vi "1_WF_Anomaly_Detection(Training).vi"() -> ()   [LabVIEW 2020]
doc: "Demonstrates the usage of Deep Learning Toolkit for solving hand written digit recognition problem with multilayer perceptron (MLP).\nDataset: MNIST http://yann.lecun.com/exdb/mnist/\nRequirements: Deep Learning Toolkit for LabVIEW"
uses:
  <vilib>/Ngene/Deep Learning Toolkit/Toolkit/NN_Layers/Layers/FC/NN_Layer_Create(FC).vi
  <vilib>/Ngene/Deep Learning Toolkit/Toolkit/Deep_Learning_Toolkit_by_Ngene.lvlib
  <vilib>/Ngene/Deep Learning Toolkit/Toolkit/NN_Activations/Controls/NN_Activation_Type.ctl
  <vilib>/Ngene/Deep Learning Toolkit/Toolkit/NN_Layers/Controls/NN_Layer_Weight_Init_Type.ctl
  <vilib>/Ngene/Deep Learning Toolkit/Toolkit/NN_Layers/Layers/FC/Controls/NN_Layer_Config(FC).ctl
  <vilib>/Ngene/Deep Learning Toolkit/Toolkit/NN_Layers/Controls/NN_Layer_Init_Params.ctl
  <vilib>/Ngene/Deep Learning Toolkit/Toolkit/NN_Network/Controls/NN_Save_Before_Destroy_Options.ctl
  <vilib>/Ngene/Deep Learning Toolkit/Toolkit/NN_Layers/Layers/Input/Controls/NN_Layer_Config(Input1D).ctl
  <vilib>/Ngene/Deep Learning Toolkit/Toolkit/NN_Layers/Layers/Input/Controls/Aug/NN_Input1D_Aug_Types.ctl
  <vilib>/Ngene/Deep Learning Toolkit/Toolkit/NN_Layers/Layers/Input/Controls/Aug/Aug_Distribution_Type.ctl
  <vilib>/Ngene/Deep Learning Toolkit/Toolkit/NN_Layers/Layers/Input/Controls/Aug/NN_Input1D_Aug_Config.ctl
  <vilib>/Ngene/Deep Learning Toolkit/Toolkit/NN_Layers/Layers/Input/Controls/NN_Layer_Config_Aug(Input1D).ctl
  <vilib>/Ngene/Deep Learning Toolkit/Toolkit/NN_Layers/Layers/BatchNorm/Controls/NN_BN_Params.ctl
  <vilib>/Ngene/Deep Learning Toolkit/Toolkit/NN_Data/Controls/NN_Data_type.ctl
  <vilib>/Ngene/Deep Learning Toolkit/Toolkit/NN_Train/Loss_Functions/NN_Set_Loss(MSE).vi
  <vilib>/Ngene/Deep Learning Toolkit/Toolkit/NN_Network/API/NN_Set_Input/1D/NN_Set_Input(1D_SGL_idx).vi
  <vilib>/Ngene/Deep Learning Toolkit/Toolkit/NN_Train/SubVIs/Dataset_Checks/NN_Check_Dataset(In1D_Out1D).vi
  <vilib>/Ngene/Deep Learning Toolkit/Toolkit/NN_Data/subVIs/Get_Data_Vals/2D/NN_Data_Get_ValByRef(2D_SGL_idx).vi
  <vilib>/Ngene/Deep Learning Toolkit/Toolkit/NN_Data/subVIs/Dataset/NN_Variant_to_DVR/2D/NN_Data_Variant_to_DVR(2D_SGL).vi
  <vilib>/Ngene/Deep Learning Toolkit/Toolkit/NN_Layers/Layers/Input/NN_Layer_Create(Input1D).vi
  <vilib>/Ngene/Deep Learning Toolkit/Toolkit/NN_Train/Controls/NN_Train_Params.ctl
  <vilib>/Ngene/Deep Learning Toolkit/Toolkit/NN_Train/Controls/NN_Train_Optimizer.ctl
  <vilib>/Ngene/Deep Learning Toolkit/Toolkit/NN_Train/Controls/NN_Train_Data_Sampling.ctl
  <vilib>/Ngene/Deep Learning Toolkit/Toolkit/NN_Train/Controls/NN_LR_Policy_Cfg.ctl
  <vilib>/Ngene/Deep Learning Toolkit/Toolkit/NN_Train/Controls/NN_LR_Policy_Type.ctl
  <vilib>/Ngene/Deep Learning Toolkit/Toolkit/NN_Train/Controls/NN_Train_Session_Data.ctl
  <vilib>/Ngene/Deep Learning Toolkit/Toolkit/NN_Network/Controls/NN_Device.ctl
panel:
  in  "Normal/Abnormal":bool
  in  "Validation(Abnormal) dataset path":path=path "D:/working/Anomaly Detection/Validation/Abnormal"
  in  "Validation(Normal) dataset path":path=path "D:/working/Anomaly Detection/Validation/Normal"
  in  "Train(Normal) dataset path":path=path "D:/working/Anomaly Detection/Train/Normal"
  out "Anomaly Score":sgl[](graph)=[0.047715902, 0.0025810003, 0.03008771, 0.04086566, 0.019934595, 0.02072841, 0.0149457455, 0.08990282, 0.04745221, 0.015019298, 0.018292785, 0.0050038695, 0.002488315, 0.0028447509, 0.004739225, 0.010417283, 0.0008608699, 0.025781095, 0.041939437, 0.002177596, 0.030179203, 0.0060115457, 0.04382831, 0.008363903, 0.035011828, 0.017032087, 0.029628694, 0.021256387, 0.014783263, 0.0030152798, 0.04009849, 0.015383124, 0.02279979, 0.09830141, 0.05799836, 0.0716297, 0.059378862, 0.07344711, 0.014608145, 0.045564353, 0.03737527, 0.0685637, 0.011108518, 0.055187643, 0.06568843, 0.046909392, 0.08090776, 0.029245019, 0.07148337, 0.11219716, 0.044215024, 0.11832294, 0.08198395, 0.053228647, 0.07091209, 0.0885334, 0.058026433, 0.017299205, 0.10348101, 0.013669521, 0.03535597, 0.10071623, 0.071124, 0.0867627, 0.055037647, 0.07809419, 0.063929304, 0.09206711, 0.03949539, 0.06335864, 0.025317574, 0.044594247, 0.08671756, 0.04539752, 0.06144145, 0.08248095, 0.05114709, 0.05862011, 0.06603286, 0.09389028, 0.06712115, 0.020853668, 0.08240548, 0.014169961, 0.06548619, 0.04012689, 0.02436462, 0.01728043, 0.069858015, 0.051284492, 0.035428643, 0.034920096, 0.05079633, 0.013650358, 0.038449407, 0.072441995, 0.01997292, 0.01657921, 0.079446375, 0.047097266, 0.10212082, 0.069970906, 0.03263557, 0.011909723, 0.02189827, 0.055327, 0.04355514, 0.028891742, 0.01913482, 0.058493435, 0.011139393, 0.01143378, 0.014839649, 0.040195167, 0.009240687, 0.010291278, 0.015378237, 0.016267061, 0.003749907, 0.02106136, 0.016822755, 0.0022764802, 0.0017397404, 0.020062983, 0.018739343, 0.05193913, 0.03168899, 0.020839095, 0.027151585, 0.03018701, 0.08075106, 0.056096375, 0.016889036, 0.014461637, 0.007615447, 0.096250534, 0.031947672, 0.045618832, 0.02684486, 0.032492936, 0.10601777, 0.045766532, 0.04348582, 0.042030573, 0.023353934, 0.05998373, 0.0366776, 0.06305903, 0.056597233, 0.063667536, 0.07347995, 0.07877654, 0.06869215, 0.030154347, 0.026351511, 0.07292321, 0.048226207, 0.06911442, 0.061527252, 0.049791813, 0.022428751, 0.09012309, 0.05610344, 0.04756078, 0.10269791, 0.044763505, 0.037158728, 0.0665781, 0.0756947, 0.09361246, 0.06363701, 0.008728512, 0.09949104, 0.07122695, 0.05130792, 0.09140627, 0.12899953, 0.076311275, 0.0602033, 0.03847994, 0.08415595, 0.026524559, 0.040219232, 0.029841065, 0.019441903, 0.027596563, 0.036504567, 0.068241, 0.040837616, 0.060942143, 0.07109749, 0.087195516, 0.055428743, 0.034413338, 0.060889006, 0.01936555, 0.07435298, 0.021365583, 0.038746476, 0.010917008, 0.096129775, 0.0073545575, 0.018815577, 0.015265167, 0.00051921606, 0.0005454421, 0.032729268, 0.07274318, 0.021330833, 0.003663838, 0.024942815, 0.02740407, 0.022603393, 0.0010912418, 0.004935682, 0.015568614, 0.02322489, 0.061240435, 0.03903711, 0.018600821, 0.029732943, 0.010967314, 0.0050938725, 0.015568972, 0.01381135, 0.0060880184, 0.051804125, 0.029231787, 0.043424904, 0.037299037, 0.031615973, 0.025720596, 0.010907292, 0.06714964, 0.0299322, 0.028302133, 0.037716627, 0.07724661, 0.07695699, 0.061065674, 0.04031396, 0.03340876, 0.020174026, 0.021361232, 0.031035602, 2.5510788e-05, 0.06611949, 0.065181196, 0.07024175, 0.07379931, 0.02338016, 0.025277913, 0.0055065155, 0.060077965, 0.05007845, 0.0006414056, 0.008725882, 0.06499711, 0.06931132, 0.09831908, 0.03877449, 0.06776312, 0.054472774, 0.063369066, 0.10040367, 0.038953096, 0.0059058666, 0.079504, 0.06579788, 0.08279285, 0.06685422, 0.040227413, 0.07007362, 0.023337401, 0.029114477, 0.057252172, 0.059272468, 0.03851404, 0.042808067, 0.045550957, 0.025526091, 0.034937397, 0.07195531, 0.025468454, 0.048014283, 0.052251175, 0.04166785, 0.056905627, 0.033443123, 0.09689638, 0.04616779, 0.0030216873, 0.031601846, 0.0032452047, 0.06213686, 0.009469092, 0.009331822, 0.017578483, 0.0055819154, 0.039248586, 0.019154549, 0.013008833, 0.014207482, 0.011167049, 0.0221982, 0.008898735, 0.017789245, 0.0074011683, 0.007955074, 0.06367123, 0.04036933, 5.1558018e-05, 0.0071540475, 0.00062155724, 0.06258881, 0.037797153, 0.0061836243, 0.02504605, 0.049601614, 0.026825964, 0.04358393, 0.02686894, 0.029046476, 0.022919714, 0.020350873, 0.035184503, 0.044800043, 0.04430455, 0.044790626, 0.050938547, 0.02782923, 0.017992377, 0.008529186, 0.06955361, 0.014567971, 0.06049311, 0.051484466, 0.07520199, 0.026690483, 0.0007273555, 0.06006384, 0.035137475, 0.023988783, 0.04264629, 0.08530253, 0.013767004, 0.012914777, 0.02451408, 0.026325583, 0.032611787, 0.064222634, 0.024199843, 0.039880395, 0.103859544, 0.014500618, 0.04841256, 0.067343056, 0.0752911, 0.06550676, 0.08130729, 0.01691103, 0.064186096, 0.030386895, 0.06907874, 0.0639095, 0.0068291724, 0.055976212, 0.021428794, 0.0060348213, 0.07295263, 0.0783522, 0.05744706, 0.0002130419, 0.040154114, 0.04585275, 0.05419886, 0.028338127, 0.08427024, 0.0041232556, 0.0687013, 0.017003741, 0.000155963, 0.07071774, 0.09512867, 0.062037416, 0.011336282, 0.040281475, 0.029887855, 0.014321253, 0.022058427, 0.014215231, 0.0059666634, 0.029912263, 0.015743941, 0.04712984, 0.016992033, 0.014030933, 0.06364295, 0.014751732, 0.03660071, 0.014532447, 0.015742123, 0.022628248, 0.018354058, 0.03808874, 0.0030311942, 0.010040998, 0.028261065, 0.017250061, 0.026884079, 0.011155605, 0.008957207, 0.008917749, 0.010064304, 0.00031030178, 0.0019487143, 0.023727417, 0.0073465705, 0.06893164, 0.04322183, 0.018407762, 0.014500916, 0.009902358, 0.03955823, 0.044618487, 0.0144174695, 0.010543764, 0.059186935, 0.04768741, 0.0011883378, 0.017390609, 0.004475951, 0.0034196973, 0.020150483, 0.017876565, 0.0039088726, 0.07626921, 0.0007389188, 0.01714021, 0.05900985, 0.033863187, 0.014671922, 0.046043932, 0.010165513, 0.011143982, 0.052004993, 0.014238179, 0.03479117, 0.025385618, 0.008669257, 0.005661547, 0.031372964, 0.054353297, 0.05981648, 0.014439642, 0.044225216, 0.009740174, 0.06296551, 0.014956772, 0.06298792, 0.05486363, 0.028136253, 0.03962207, 0.039901912, 0.058602363, 0.041279078, 0.040257484, 0.013936877, 0.07086399, 0.02723828, 0.03215918, 0.044406503, 0.02660507, 0.09844187, 0.015807092, 0.0022975206, 0.018990919, 0.03249289, 0.052985646, 0.0596376, 0.018778317, 0.05455137, 0.038281374, 0.022315275, 0.053559072, 0.046947896, 0.0041363873, 0.022759922, 0.040063687, 0.02208151, 0.024711475, 0.0038131028, 0.0016301423, 0.019919693, 0.073530674, 0.012975574, 0.0032351613, 0.033508807, 0.022399366, 0.0033747852, 0.028906435, 0.034864515, 0.00394547, 0.0149511695, 0.00368917, 0.02648884, 0.0371809, 0.017273486, 0.00536865, 0.04249835, 0.024990976, 0.014424562, 0.0037795901, 0.035405636, 0.054773033, 0.023358285, 0.023425102, 0.0194816, 0.0021141171, 0.033955276, 0.031220973, 0.016408503, 0.04635465, 0.053446114, 0.03696829, 0.03385341, 0.014172077, 0.0044620037, 0.02061069, 0.07261884, 0.008972824, 0.015659451, 0.008246541, 0.0019729137, 0.0710991, 0.05038321, 0.0028544068, 0.037355185, 0.03963381, 0.014549613, 0.0038695335, 0.03834486, 0.0026820302, 0.029096782, 0.03855908, 0.041218698, 0.02275443, 0.04536414, 0.066978574, 0.051580906, 0.0017378926, 0.025789797, 0.040744185, 0.009256244, 0.034905314, 0.03186083, 0.05465746, 0.08973676, 0.04353434, 0.022286654, 0.0051453114, 0.00048309565, 0.03697884, 0.04100603, 0.006838441, 0.035681367, 0.012636542, 0.045780897, 0.04042518, 0.0755156, 0.0016447008, 0.0059679747, 0.0072202384, 0.01067698, 0.0070519447, 0.038136035, 0.0004273653, 0.06682205, 0.01769942, 0.06582381, 0.029339477, 0.01768677, 0.0058039725, 0.023210868, 0.023157693, 0.0009084493, 0.016897243, 0.005831221, 0.031396866, 0.01948181, 0.04044591, 0.017842405, 0.013730571, 0.021805942, 0.01105006, 0.02152425, 0.065292746, 0.021284014, 0.024479747, 0.008365303, 0.023296893, 0.0356026, 0.0074109435, 9.998679e-05, 0.0040650666, 0.06386435, 0.016895354, 0.017855644, 0.011718214, 0.003956735, 0.062547326, 0.054714262, 0.014458597, 0.002638638, 0.010711074, 0.038244665, 0.007031977, 0.017196178, 0.044457376, 0.03590107, 0.009813726, 0.019953907, 0.047487378, 0.019844353, 0.034417152, 0.018498003, 0.014561772, 0.06384802, 0.031535804, 0.011589706, 0.001119554, 0.04682505, 0.056577682, 0.00937444, 0.0059499145, 0.0002413392, 0.03447455, 0.027209401, 0.00010806322, 0.029770195, 0.0073183775, 0.04158777, 0.011110187, 0.026478708, 0.0050107837, 0.04203552, 0.012228727, 0.007688701, 0.004582584, 0.025569081, 0.042006016, 0.032153547, 0.020944834, 0.05830443, 0.024040341, 0.04531777, 0.005422652, 0.055900514, 0.06162244, 0.048154175, 0.037574172, 0.009326458, 0.028306842, 0.039817393, 0.025396824, 0.00022929907, 0.019289196, 0.037306607, 0.0028678775, 0.02366358, 0.072078794, 0.032467306, 0.0025970936, 0.017390937, 0.010368198, 0.002228558, 0.022588015, 0.017153263, 0.03150198, 0.0044680536, 0.008227289, 0.005346477, 0.0020497143, 0.041761637, 0.009586662, 0.042886183, 0.035135306, 0.016337283, 0.043457747, 0.03837393, 0.051611952, 0.021941999, 0.014178699, 0.037345707, 0.014388442, 0.018260948, 0.05853848, 0.029040098, 0.025413066, 0.012405887, 0.022361755, 0.026380628, 0.018216312, 0.0015644729, 0.020917326, 0.019475996, 0.024011612, 0.017211854, 0.021681547, 0.015715957, 0.027698696, 0.011981189, 0.03608662, 0.0057917833, 0.009307146, 0.009901524, 0.0032221675, 0.037121236, 0.006166756, 0.0054784417, 0.011930764, 0.0014172792, 0.05286801, 0.044288397, 0.011786461, 0.005430579, 0.019859195, 0.013941109, 0.034538627, 0.0028657913, 0.047690094, 0.0014411211, 0.06301719, 0.01045537, 0.036057293, 0.0025453568, 0.009298801, 0.028163493, 0.02333951, 0.0074952245, 0.0109013915, 0.037617683, 0.021433711, 0.015725017, 0.02000618, 0.018161058, 0.0010209084, 0.004538834, 0.01497376, 0.008681357, 0.03325498, 0.012607813, 0.025254905, 0.046028495, 0.020547867, 0.027874947, 0.019095242, 0.0067641735, 0.029079497, 0.0304721, 0.03780067, 0.042236805, 0.03193754, 0.009736061, 0.045875132, 0.019194245, 0.020226657, 0.012554288, 0.024856985, 0.0032795072, 0.008099079, 0.016595662, 0.009702802, 0.043530464, 0.055282056, 0.008933961, 0.06304589, 0.025927782, 0.0014396906, 0.02054578, 0.024381757, 0.037120134, 0.057779104, 0.032738894, 0.043530256, 0.01557222, 0.025099546, 0.01085031, 0.003905654, 0.012544721, 0.048828557, 0.02195388, 0.020418592, 0.005827032, 0.040778756, 0.014163524, 0.015930746, 0.029816426, 0.0112039, 0.020876735, 0.015639842, 0.046031654, 0.006152123, 0.009709865, 0.015743494, 0.02742067, 0.014137089, 0.019241929, 0.041894466, 0.0380778, 0.017151564, 0.028223097, 0.0073495805, 0.02557528, 0.05750835, 0.052480698, 0.023915052, 0.018465817, 0.0607692, 0.04103142, 0.0051792264, 0.062756956, 0.0017514229, 0.047276914, 0.03923863, 0.0414052, 0.02587217, 0.0129439235, 0.0024460554, 0.030288875, 0.006010711, 0.012355745, 0.020411193, 0.021352828, 0.015683293, 0.00407207, 0.016973317, 0.03465146, 0.054066658, 0.016430616, 0.00036644936, 0.06764871, 0.0023283362, 0.026587725, 0.010902405, 0.015266538, 0.019437015, 0.029160678, 0.01953113, 0.0073716044, 0.048199713, 0.008838415, 0.008901656, 0.011385918, 0.030213773, 0.022456944, 0.016247928, 0.014270544, 0.008595407, 0.061956167, 0.0069187284, 0.017821848, 0.039972365, 0.0042414665, 0.05832219, 0.054510415, 0.026431322, 0.035200596, 0.02948153, 0.06208718, 0.032461464, 0.038664818, 0.0013316274, 0.02666688, 0.009301305, 0.0017058849, 0.0044255257, 0.010630608, 0.0064505935, 0.03288746, 0.029383928, 0.0012662113, 0.074050486, 0.061786264, 0.04708299, 0.028854996, 0.07325849, 0.03170407, 0.01122728, 0.021617055, 0.027222857, 0.027592361, 0.07195831, 0.030459575, 0.033628687, 0.021496147, 0.04374882, 0.018187447, 0.036165297, 0.023571942, 0.021791894, 0.0085014105, 0.0108578205, 0.05386503, 0.05539906, 0.0006233007, 0.0037605017, 0.0017763972, 0.022153169, 0.062341124, 0.044531137, 0.068103254, 0.06815606, 0.004120916, 0.022712916, 0.016933113, 0.025369227, 0.04291123, 0.040973663, 0.0039020777, 0.059156835, 0.011050403, 0.06237316, 0.03736663, 0.044977903, 0.015730858, 0.014122486, 0.016065955, 0.029520154, 0.03648597, 0.07051659, 0.0013179779, 0.02324748, 0.065591395, 0.025277019, 0.004920244, 0.022859454, 0.00853914, 0.03705609, 0.019424379, 0.025880516, 0.026400805, 0.0066967607, 0.0113399625, 0.022522569, 0.024003327, 0.017210007, 0.024513185, 0.043397844, 0.014945388, 0.005337, 0.02035439, 0.005132377, 0.034187138, 0.0031021833, 0.037469983, 0.0021530986, 0.0030584931, 0.00672853, 0.013904095, 0.026868641, 0.006538272, 0.028280377, 0.01350528, 0.028854728, 0.027126312, 0.0120072365, 0.05255574, 0.0076737404, 0.036070883, 0.006802559, 0.01700586, 0.031392276, 0.016890705, 0.03442079, 0.018255591, 0.051992595, 0.0022095442, 0.03269446, 0.022119522, 0.050598025, 0.04284787, 0.016165614, 0.046081275, 0.04473442, 0.037802935, 0.03842947, 0.06306109, 0.02220431, 0.028944224, 0.0045770705, 0.042494506, 0.008256197, 0.046750844, 0.0036908686, 0.02311422, 0.00077693164, 0.0039515197, 0.018653229, 0.07726545, 0.040283788, 0.059524216, 0.009495227, 0.047083277, 0.020730667, 0.049935937, 0.012333117, 0.05908279, 0.06908634, 0.06223628, 0.033225983, 0.004655093, 0.05483687, 0.056556523, 0.016717672, 0.02827838, 0.071347386, 0.01589346, 0.06992328, 0.0028676689, 0.0745683, 0.08355194, 0.040931225, 0.06754261, 0.021474183, 0.027969003, 0.0076584816, 0.047234952, 0.019856632, 0.01673466, 0.048998177, 0.027508855, 0.002669096, 0.024096966, 0.023823977, 0.030286014, 0.053969204, 0.01939392, 0.023516238, 0.031034708, 0.038506985, 0.047025442, 0.018635392, 0.034413576, 0.012740314, 0.050352156, 0.018050969, 0.041873693, 0.0032143593, 0.00026267767, 0.045363843, 0.011178076, 0.020819843, 0.020995736, 0.019217253, 0.024541855, 0.021695912, 0.042124867, 0.039527237, 0.013458908, 0.022761524, 0.042527378, 0.018703818, 0.016821265, 0.007864118, 0.018794596, 0.002880156, 0.011899173, 0.03275305, 0.051254213, 0.019226491, 0.01218617, 0.02842462, 0.06131518, 0.037252605, 0.0028996468, 0.004270494, 0.023361921, 0.011644244, 0.0009986758, 0.011639357, 0.022646487, 0.030133486, 0.0023872852, 0.05259055, 0.02781564, 0.019533455, 0.011627108, 0.05079347, 0.03150606, 0.006302446, 0.0426268, 0.058501363, 0.041143566, 0.05102235, 0.017350227, 0.044205993, 0.059088513, 0.016211674, 0.013123974, 0.10360771, 0.06259384, 0.07653545, 0.054447174, 0.06402078, 0.05027257, 0.010026, 0.0012903884, 0.017136708, 0.031048805, 0.02365224, 0.028259784, 0.034087062, 0.09500918, 0.10728651, 0.08586332, 0.15200752, 0.11835763, 0.16687855, 0.17173398, 0.19207877, 0.24995285, 0.19854617, 0.1764394, 0.21960711, 0.20500982, 0.24628907, 0.25381434, 0.28048664, 0.27028018, 0.2936979, 0.31636304, 0.34905374, 0.2980923, 0.33609152, 0.34724927, 0.36034995, 0.32336485, 0.3780651, 0.39284462, 0.34902, 0.36514992, 0.36266762, 0.39584345, 0.41756094, 0.40966296, 0.41349822, 0.38569427, 0.40935284, 0.41609186, 0.450463, 0.41314453, 0.4588943, 0.4453857, 0.4970355, 0.40337288, 0.482355, 0.4416746, 0.42152506, 0.44260156, 0.47098666, 0.5108878, 0.48012918, 0.44878733, 0.4477948, 0.42475057, 0.45093548, 0.45039457, 0.47215348, 0.44049102, 0.40422547, 0.47909123, 0.3841099, 0.44589847, 0.38989443, 0.37071013, 0.38811028, 0.34597635, 0.43548524, 0.3414498, 0.3586625, 0.34691823, 0.32170552, 0.3432048, 0.3056975, 0.32426786, 0.34024483, 0.2951817, 0.2671197, 0.26881975, 0.26968446, 0.2301977, 0.20990345, 0.2044313, 0.23516709, 0.22842091, 0.19398198, 0.15870875, 0.18524614, 0.15944, 0.12737198, 0.14472875, 0.13780338, 0.11759119, 0.11801046, 0.12755883, 0.08333115, 0.04292041, 0.0053507686, 0.090944454, 0.011543207, 0.019948155, 0.005117163, 0.052084804, 0.019741476, 0.054212824, 0.04441881, 0.13271424, 0.07727906, 0.07064524, 0.11240524, 0.11976227, 0.15400401, 0.17976153, 0.11758286, 0.17170012, 0.16568577, 0.16813141, 0.22549754, 0.20982617, 0.30876273, 0.29224867, 0.29248106, 0.25594628, 0.30639195, 0.25497818, 0.29515803, 0.33552432, 0.31921124, 0.3067137, 0.24702018, 0.31533587, 0.3658582, 0.36704057, 0.35608792, 0.37667185, 0.39209074, 0.38716066, 0.36213583, 0.37161422, 0.39183903, 0.40344232, 0.45020974, 0.40157467, 0.43283337, 0.45464092, 0.4650002, 0.4078399, 0.44429886, 0.39547884, 0.43432665, 0.42246765, 0.37123108, 0.45490205, 0.47389477, 0.41789138, 0.4096067, 0.42737395, 0.40034485, 0.46786267, 0.4371156, 0.4394366, 0.42294914, 0.40482736, 0.45386964, 0.41958004, 0.41875392, 0.43256062, 0.41303563, 0.39032292, 0.35937828, 0.39335245, 0.37966162, 0.3207494, 0.34534585, 0.31439143, 0.35419393, 0.35136044, 0.2714697, 0.3071317, 0.3122294, 0.3169033, 0.25213546, 0.17343307, 0.28683865, 0.21691835, 0.2296286, 0.24889404, 0.16115963, 0.22275573, 0.21703765, 0.16188416, 0.20319314, 0.1351986, 0.06677234, 0.1281872, 0.121130824, 0.095688134, 0.1242291, 0.053609952, 0.076433584, 0.05226974, 0.019035295, 0.04608327, 0.051075764, 0.041780293, 0.002134502, 0.016285017, 0.014686391, 0.035825074, 0.07825789, 0.08928537, 0.0548864, 0.06708887, 0.12011245, 0.15190464, 0.18970129, 0.18528613, 0.14642143, 0.17787713, 0.19936293, 0.18542993, 0.20661956, 0.19919503, 0.20683569, 0.2254808, 0.23557454, 0.26535833, 0.278089, 0.33645636, 0.32736862, 0.33491045, 0.39516985, 0.3846696, 0.3192271, 0.35689765, 0.38337123, 0.36489803, 0.37651008, 0.3748414, 0.393134, 0.39248073, 0.4201432, 0.3958295, 0.40006888, 0.44861025, 0.42295724, 0.42890185, 0.43160933, 0.45493543, 0.42765456, 0.45452338, 0.4304362, 0.3685441, 0.40631235, 0.40755337, 0.44663572, 0.42920858, 0.4233718, 0.38530934, 0.4663105, 0.44680423, 0.41557652, 0.4176917, 0.41162497, 0.39407736, 0.3614812, 0.4195885, 0.43954504, 0.398023, 0.42228526, 0.35042423, 0.41396052, 0.387394, 0.34367543, 0.39515483, 0.3506348, 0.31913853, 0.2936976, 0.31444108, 0.33919525, 0.34410495, 0.30420256, 0.31221074, 0.29192054, 0.26789325, 0.28812188, 0.24974829, 0.28794038, 0.19300196, 0.18817458, 0.22424757, 0.21683434, 0.17423075, 0.18689865, 0.15911564, 0.1098187, 0.1137068, 0.1202703, 0.122633025, 0.0856407, 0.08053285, 0.061647743, 0.057097957, 0.04922293, 0.05724816, 0.001163342, 0.003945347, 0.013643123, 0.010027081, 0.0108757615, 0.08470482, 0.08373572, 0.07757519, 0.11199492, 0.12700078, 0.095326394, 0.101403326, 0.11915606, 0.12910521, 0.14894515, 0.14079827, 0.18173847, 0.21615872, 0.21829468, 0.20423907, 0.26865637, 0.2269032, 0.2324276, 0.28228277, 0.24751759, 0.24826968, 0.24185771, 0.32894927, 0.27344245, 0.280459, 0.3615561, 0.30175394, 0.41692477, 0.39269507, 0.4353841, 0.4031086, 0.3606316, 0.32949835, 0.35444605, 0.3942849, 0.36237657, 0.4052484, 0.37975264, 0.4004873, 0.40951306, 0.37155914, 0.39112228, 0.4454437, 0.39413953, 0.50151587, 0.41670054, 0.40516222, 0.42869157, 0.3719684, 0.45527446, 0.4354626, 0.3855487, 0.37958026, 0.44542348, 0.4463405, 0.41590822, 0.4122483, 0.369613, 0.43961388, 0.4128676, 0.41172755, 0.34417838, 0.35851038, 0.39117116, 0.39790213, 0.37138748, 0.35669726, 0.3281142, 0.2862726, 0.37756056, 0.33414364, 0.34650546, 0.29717416, 0.27725822, 0.3376863, 0.2689234, 0.2523632, 0.29676956, 0.23450476, 0.23432785, 0.19972146, 0.15833294, 0.19368213, 0.17604354, 0.19002718, 0.19075039, 0.19072005, 0.16317034, 0.125684, 0.1071043, 0.10264088, 0.15311924, 0.094702795, 0.104200944, 0.06759892, 0.044868685, 0.04457221, 0.044390526, 0.041599587, 0.009926207, 0.016707115, 0.041193113, 0.0037209839, 0.0052166283, 0.098388866, 0.061579272, 0.068443745, 0.14088993, 0.095683336, 0.12377456, 0.11309707, 0.10020709, 0.1467542, 0.14300224, 0.21611425, 0.19595557, 0.22386393, 0.23261929, 0.26708806, 0.21489549, 0.265872, 0.28999883, 0.2594192, 0.30382723, 0.27976763, 0.29174453, 0.3503322, 0.29209417, 0.32555664, 0.33462924, 0.3401587, 0.3462242, 0.35842872, 0.34520954, 0.38784915, 0.35780674, 0.04020959, 0.08372176, 0.0776189, 0.060139894, 0.097709894, 0.08003843, 0.07797986, 0.051816642, 0.047575057, 0.069582105, 0.0674656, 0.07808864, 0.05615127, 0.06218505, 0.017017365, 0.06487441, 0.0010330677, 0.038105726, 0.011226773, 0.021775484, 0.07733595, 0.063058734, 0.053465366, 0.027271926, 0.046481013, 0.09432882, 0.038227737, 0.07192367, 0.06956929, 0.051414967, 0.02923429, 0.046415985, 0.06561458, 0.05245942, 0.018404424, 0.051792502, 0.049830258, 0.033891737, 0.07359338, 0.005530715, 0.07115489, 0.029260635, 0.041643023, 0.018743515, 0.015555918, 0.011587262, 0.03343004, 0.03461951, 0.021687478, 0.03833261, 0.037670672, 0.007627785, 0.03832051, 0.009793431, 0.014735758, 0.016792923, 0.024642855, 0.025508285, 0.030881107, 0.06366445, 0.030663773, 0.03541994, 0.02178897, 0.036904372, 0.05318751, 0.0036119688, 0.010256409, 0.009168476, 0.015120845, 0.0044179335, 0.03668298, 0.047770068, 0.0040861666, 0.015399441, 0.026566625, 0.014979377, 0.012833685, 0.03807065, 0.015267134, 0.014687568, 0.015760303, 0.07911828, 0.0031440854, 0.0021149516, 0.056374997, 0.05004096, 0.012219667, 0.10929704, 0.057184935, 0.0428949, 0.012614727, 0.08175272, 0.031056225, 0.04383546, 0.06013894, 0.05104482, 0.04815787, 0.031544924, 0.06282681, 0.082015455, 0.06751734, 0.07721686, 0.06628597, 0.06583208, 0.0514853, 0.03862065, 0.028685391, 0.053161442, 0.032678843, 0.050779343, 0.026046753, 0.0924958, 0.090927124, 0.07286954, 0.08844817, 0.07528716, 0.094216466, 0.09988135, 0.08372027, 0.053912878, 0.06538564, 0.08065671, 0.10297024, 0.036806226, 0.035205603, 0.055594742, 0.076091886, 0.038747013, 0.10293436, 0.054749668, 0.045713365, 0.06508398, 0.04049349, 0.09987658, 0.015277386, 0.058148026, 0.11515927, 0.042001188, 0.0035157204, 0.062142074, 0.03937179, 0.098088264, 0.05230272, 0.05701375, 0.00393641, 0.0011408925, 0.05078411, 0.016378462, 0.04868883, 0.08481455, 0.047059596, 0.022682726, 0.026164562, 0.012143731, 0.040976644, 0.017727047, 0.09220639, 0.020482719, 0.061356157, 0.0021803975, 0.0037044883, 0.009715736, 0.052236304, 0.023337841, 0.025850326, 0.050537787, 0.013436541, 0.0055997074, 0.03712785, 0.0077945627, 0.05592349, 0.0012027062, 0.013075605, 0.020720191, 0.024010241, 0.01479581, 0.016827404, 0.030558363, 0.015124962, 0.03727129, 0.0035442412, 0.027584583, 0.006701201, 0.013814449, 0.03564605, 0.0070546865, 0.013096958, 0.011903524, 0.032976568, 0.056175947, 0.025060475, 0.031738818, 0.07220447, 0.09542501, 0.039100826, 0.07739991, 0.07337773, 0.008980811, 0.0033184886, 0.06001824, 0.055814266, 0.047296286, 0.029973269, 0.056255817, 0.059824467, 0.07536459, 0.10366714, 0.07212579, 0.039361894, 0.080531, 0.09450114, 0.063426554, 0.06223941, 0.064344406, 0.071787834, 0.108517885, 0.105495214, 0.13214654, 0.038695037, 0.0952819, 0.1254859, 0.11156398, 0.09407437, 0.09940964, 0.0997901, 0.07735628, 0.104536176, 0.10556692, 0.085997224, 0.06963652, 0.08141792, 0.07232982, 0.09118146, 0.09753454, 0.084991515, 0.084968925, 0.10546726, 0.044424415, 0.06955904, 0.091522336, 0.029014528, 0.087307155, 0.07887232, 0.10404587, 0.0933848, 0.05388266, 0.073718905, 0.05041969, 0.09238088, 0.07978207, 0.054448187, 0.087059855, 0.042691827, 0.04288125, 0.09604609, 0.04231757, 0.03933978, 0.044936746, 0.06721625, 0.09342125, 0.021906376, 0.072917074, 0.06430268, 0.0135733485, 0.009343535, 0.02072157, 0.03508824, 0.073774785, 0.01874414, 0.07625115, 0.01645761, 0.022751573, 0.01261903, 0.035796292, 0.023246653, 0.023820166, 0.043936133, 0.0059004873, 0.04301019, 0.008450046, 0.00059069693, 0.01853396, 0.027813554, 0.012709439, 0.00031155348, 0.04911858, 0.051597416, 0.025631398, 0.044952452, 0.0067074895, 0.087528706, 0.055566102, 0.05398935, 0.037686825, 0.021915913, 0.032868624, 0.0063841343, 0.06768656, 0.05494052, 0.014489055, 0.06333095, 0.057601333, 0.037834942, 0.106841505, 0.020667076, 0.06850928, 0.040855587, 0.08487272, 0.08369887, 0.1063323, 0.09598112, 0.03803581, 0.10189116, 0.042521775, 0.10309875, 0.059610844, 0.080476224, 0.08484912, 0.15615201, 0.094754815, 0.094225824, 0.061502397, 0.12885815, 0.14350593, 0.087043405, 0.08951622, 0.109604, 0.09813243, 0.095102966, 0.1376431, 0.13674217, 0.0778563, 0.11322141, 0.15300399, 0.06646758, 0.15084398, 0.12895566, 0.13326317, 0.15391177, 0.08805472, 0.090057015, 0.13663888, 0.09571856, 0.108368516, 0.09767032, 0.1320008, 0.061623037, 0.09587866, 0.05944717, 0.11934781, 0.113535106, 0.09484959, 0.111512065, 0.053406477, 0.106235206, 0.121563554, 0.15173966, 0.11799276, 0.09788814, 0.037851036, 0.0565719, 0.042096704, 0.058404982, 0.07150829, 0.06508112, 0.103627235, 0.013689637, 0.04077673, 0.0649703, 0.0070453137, 0.07181531, 0.016764373, 0.06798321, 0.016805626, 0.025288634, 0.02255059, 0.018744105, 0.022342317, 0.022829836, 0.021267038, 0.016382612, 0.0014830977, 0.03296882, 0.052188113, 0.029418543, 0.05269873, 0.06283882, 0.046594918, 0.021034151, 0.032283366, 0.029017746, 0.036972046, 0.00626719, 0.0050839484, 0.053715378, 0.03149569, 0.032604814, 0.060468495, 0.04465568, 0.06333661, 0.08593392, 0.07434738, 0.040181577, 0.09658438, 0.05523789, 0.052340746, 0.09991956, 0.08627689, 0.016836047, 0.07450122, 0.045303702, 0.06741166, 0.078064024, 0.14879322, 0.10289347, 0.08531064, 0.04481536, 0.05656004, 0.073052704, 0.04151666, 0.10891342, 0.084085464, 0.076387286, 0.102749705, 0.096190035, 0.099155486, 0.10787815, 0.10682976, 0.14352363, 0.133268, 0.10419649, 0.13158739, 0.1202181, 0.089677155, 0.08486706, 0.05886233, 0.14240217, 0.17081511, 0.18490946, 0.11767632, 0.11474764, 0.093085706, 0.06527203]
  out "Loss Chart":sgl(graph)=6.871157
  out "Input & Reconstructed Signals":sgl[][](graph)=[[-203.69182, -196.45944, -206.42105, -212.12776, -209.98431, -212.81482, -214.06697, -234.45668, -226.42854, -220.56462, -214.24974, -221.52092, -221.16281, -222.03725, -222.54259, -226.90015, -224.91339, -219.17255, -215.53453, -224.83737, -217.877, -226.08276, -213.40121, -224.96735, -213.59717, -216.4723, -226.23088, -212.33847, -211.97202, -214.08366, -201.33636, -212.25195, -211.15195, -179.20767, -185.76039, -179.36887, -178.70908, -171.73268, -182.25404, -170.74457, -168.62994, -156.8247, -171.38605, -150.91496, -143.59477, -143.30174, -130.10214, -137.22119, -121.803986, -106.51268, -117.308395, -93.7625, -96.723854, -97.62513, -87.381096, -77.151985, -78.23366, -81.768196, -54.604557, -69.67931, -57.994568, -35.828102, -36.21024, -25.736954, -26.630962, -14.377393, -11.056967, 2.416106, -3.241106, 9.206075, 7.0362177, 18.38262, 35.452217, 32.255405, 42.825947, 54.835426, 54.0353, 62.54883, 70.807884, 84.21367, 84.26908, 79.644875, 100.897316, 91.00079, 109.55669, 109.47046, 111.927505, 116.2273, 134.60593, 135.90828, 137.86287, 143.26082, 152.59111, 148.95609, 159.94786, 173.14607, 155.76651, 169.33902, 188.98714, 185.78334, 203.069, 199.43301, 194.55254, 193.17833, 188.66443, 210.55849, 211.09325, 196.82597, 210.99236, 223.07843, 209.00655, 211.09589, 212.43848, 227.56683, 221.81776, 218.5701, 218.54922, 219.29591, 223.26003, 219.82527, 221.32254, 224.81364, 225.18246, 220.54489, 229.37744, 211.93462, 215.83464, 217.4786, 214.76361, 212.59512, 199.01974, 203.01688, 210.50662, 208.68921, 207.9323, 184.01987, 196.81256, 190.41148, 191.79723, 187.0817, 165.83574, 198.66397, 173.4034, 169.67267, 169.83505, 156.7239, 157.75739, 146.86583, 143.61665, 136.87979, 129.4848, 122.93364, 119.83389, 123.56296, 118.95564, 102.018425, 101.94571, 91.17254, 86.75346, 83.56996, 83.8971, 61.17046, 63.095177, 58.665413, 38.7125, 46.13676, 41.241905, 27.461256, 18.55327, 7.53301, 8.007118, 14.225158, -14.277849, -14.454468, -16.393902, -32.977505, -48.719887, -42.794704, -45.88879, -47.395184, -65.07743, -45.234108, -67.73261, -71.96186, -75.94605, -84.38318, -93.0011, -106.85784, -106.52103, -117.346115, -126.0234, -135.64693, -134.0229, -134.7392, -146.61336, -132.87227, -160.64471, -153.20773, -162.41916, -160.78008, -186.03116, -165.75491, -167.56427, -180.06364, -180.35538, -184.6909, -196.25504, -209.69836, -200.7194, -198.08067, -208.06628, -211.53697, -213.26482, -210.50189, -211.45543, -211.06352, -211.38602, -233.3377, -229.6889, -225.98419, -229.8559, -221.04784, -223.17747, -221.38345, -222.04527, -224.13887, -237.793, -218.10437, -214.21802, -214.96823, -215.61217, -215.82706, -218.18225, -203.00409, -210.25627, -208.7275, -204.30801, -192.66081, -190.09033, -191.26424, -193.36465, -191.9019, -191.95824, -188.0733, -182.15146, -185.75388, -166.05133, -162.19652, -156.66197, -151.24817, -158.78876, -153.53331, -156.12155, -135.3413, -132.46117, -139.04605, -131.58578, -112.56069, -106.00528, -93.04342, -101.57413, -88.61685, -85.566536, -77.19142, -62.063118, -70.57126, -72.02259, -47.879044, -44.448505, -33.889717, -30.994986, -30.66542, -16.782331, -21.279024, -12.932525, 0.5405211, 7.985392, 9.72337, 17.713936, 25.09223, 27.006262, 36.224976, 51.829273, 47.39243, 59.52343, 67.260284, 71.20028, 81.57735, 82.42635, 104.13513, 98.20027, 92.634796, 107.18444, 104.82115, 126.51285, 119.87258, 121.12036, 133.33884, 133.30034, 149.33966, 149.79709, 147.35788, 158.9298, 163.00009, 159.79243, 167.54431, 178.50941, 180.09627, 180.49078, 201.7611, 180.63136, 193.66762, 198.99698, 200.54916, 188.49869, 197.32869, 210.52406, 217.45105, 225.74438, 209.32176, 207.21986, 225.80853, 213.82886, 216.73927, 218.3158, 215.71573, 214.12799, 214.48691, 214.61026, 213.37476, 218.68098, 220.56183, 222.353, 206.98712, 218.98369, 206.76166, 207.72372, 200.35153, 210.07428, 214.73456, 197.98468, 201.567, 201.60269, 194.24489, 181.12738, 195.17592, 192.02046, 185.63661, 181.60185, 176.25317, 164.58656, 169.87204, 161.7887, 141.8737, 158.75986, 145.82098, 136.23767, 129.29015, 126.35838, 117.04625, 127.22135, 110.11534, 112.46715, 97.4211, 92.66172, 103.63901, 82.32571, 84.37709, 84.728355, 59.291367, 51.515476, 50.052708, 57.06887, 41.00301, 32.91534, 24.192274, 23.67885, 3.2951412, 15.810419, -6.408311, -0.9608977, -3.8774314, -27.532257, -40.11088, -39.128983, -33.680706, -47.347557, -51.573086, -54.557102, -52.545975, -67.73166, -69.608, -84.45894, -87.53854, -101.311165, -100.318085, -99.11257, -123.7543, -118.02042, -129.02417, -129.48778, -127.981895, -142.47078, -146.96497, -156.9813, -153.6075, -160.32983, -169.50266, -163.13998, -178.29219, -178.83736, -178.09027, -182.17975, -190.57542, -191.92554, -195.8277, -193.02542, -200.07683, -221.50359, -197.22676, -205.82213, -209.15977, -212.42343, -226.21397, -207.93156, -216.61981, -224.05049, -208.51514, -212.23502, -224.6852, -220.94626, -224.28577, -226.42073, -230.19612, -220.82964, -225.57812, -205.6154, -223.02266, -217.88635, -206.63763, -211.23283, -214.15874, -204.70946, -211.16028, -208.52544, -196.3188, -202.74284, -194.93011, -194.06744, -194.71938, -192.08122, -182.31049, -172.9552, -167.80405, -174.61449, -163.14594, -166.86235, -149.52827, -156.49037, -139.92291, -136.83273, -138.20729, -129.9307, -124.58354, -114.57544, -112.97303, -107.458206, -107.77515, -88.11264, -92.58281, -85.1618, -75.98244, -73.77478, -50.053955, -63.4063, -60.168594, -49.442177, -39.721706, -28.083445, -19.766977, -22.613203, -7.3076715, -4.49247, -1.364334, 12.854177, 18.227495, 14.672733, 26.102383, 36.975285, 39.379562, 46.970757, 48.675144, 54.631233, 65.74073, 85.08736, 70.80586, 81.17644, 94.92211, 87.744156, 99.92995, 112.29755, 119.72748, 118.06692, 126.70828, 129.5254, 127.80268, 148.60342, 140.81436, 148.95152, 165.47961, 154.08217, 161.4181, 168.5329, 182.49736, 164.93446, 187.76599, 191.86203, 185.40442, 194.18738, 188.89073, 207.65303, 207.21805, 217.28513, 195.97293, 202.56761, 205.47517, 219.1613, 218.75089, 214.41342, 203.37148, 219.84653, 226.95827, 222.18083, 224.1665, 242.18379, 213.26804, 226.28506, 216.39476, 215.36787, 220.9081, 222.75131, 213.51723, 220.87631, 227.06323, 209.14583, 206.82751, 209.33893, 201.5126, 193.92514, 195.22058, 204.3029, 208.02956, 208.49861, 193.1385, 183.38274, 180.5134, 171.20221, 158.70317, 165.47176, 166.25119, 168.51488, 162.36406, 148.80508, 142.79855, 149.24123, 133.75647, 134.00723, 120.53258, 116.05795, 102.11626, 114.63473, 106.807686, 100.50714, 93.67752, 91.69247, 74.36735, 77.17743, 54.762703, 68.56786, 41.802284, 43.838524, 40.155174, 36.047047, 25.149393, 18.442154, 17.498028, 6.2646623, 2.200507, -10.895248, -5.4043655, -26.747019, -28.042177, -34.01534, -42.673428, -41.507984, -45.71418, -73.03026, -69.18816, -76.43514, -75.03233, -89.11125, -98.30463, -94.221375, -102.264, -107.26439, -129.56744, -115.945114, -121.47464, -128.46762, -137.74962, -157.33136, -160.49142, -156.11006, -158.07327, -165.05066, -176.21872, -173.28767, -171.79291, -190.66977, -192.69626, -190.2753, -196.54895, -206.51698, -193.71736, -193.33987, -200.28047, -203.86517, -225.32352, -204.8314, -211.77847, -216.9887, -207.16199, -206.50136, -223.76987, -221.292, -223.73792, -216.12611, -218.34973, -225.38594, -218.45515, -223.60359, -215.13895, -221.97356, -217.80511, -221.9974, -212.15147, -217.86511, -221.20528, -218.77982, -209.62341, -203.51855, -203.72314, -204.01324, -192.16695, -209.04968, -189.52373, -198.34143, -180.26387, -175.29062, -174.683, -173.3822, -176.08165, -167.20636, -160.12383, -158.78476, -160.26497, -150.6506, -141.2864, -144.51172, -134.24074, -117.10109, -121.087845, -122.496704, -113.18617, -109.11163, -106.13486, -93.93888, -89.00322, -94.440475, -79.567665, -72.18545, -68.96316, -61.69193, -44.457207, -45.4592, -30.747316, -25.887527, -31.520948, -10.45014, -4.7102566, 5.186868, 5.0260797, 9.882888, 22.40297, 16.706774, 31.502626, 47.889236, 47.529625, 53.379135, 56.977413, 65.846825, 73.53135, 78.05192, 80.53547, 91.42016, 97.31424, 93.11721, 100.74915, 116.08357, 120.651825, 115.99231, 125.52452, 142.5808, 138.04996, 146.9537, 147.62363, 155.81332, 150.93091, 166.12003, 170.51482, 176.38338, 177.49985, 194.84833, 196.62921, 192.66875, 194.74333, 201.56621, 196.81413, 211.32927, 205.23221, 220.24562, 211.54587, 198.47588, 218.0293, 226.09375, 218.50911, 223.03172, 228.75925, 217.59853, 222.12115, 227.25633, 216.09177, 220.21591, 221.82599, 230.16148, 229.47865, 224.15498, 222.59067, 219.1263, 223.60352, 212.0988, 221.66588, 210.65883, 203.75316, 217.57149, 203.55, 203.01715, 206.58339, 209.05908, 191.4067, 186.52783, 181.86317, 180.735, 182.22334, 169.46996, 181.00662, 166.98561, 164.50697, 168.68567, 158.70708, 150.93623, 151.82295, 144.88867, 126.832695, 118.49231, 128.38416, 105.34898, 120.942665, 109.06553, 97.78902, 90.62838, 81.33116, 70.13301, 69.66267, 60.59274, 60.822666, 52.05611, 48.755924, 43.702644, 34.909267, 19.481146, 19.211067, 12.619537, 9.401513, 13.626902, -6.279246, -13.66338, -23.715942, -26.208935, -35.250416, -40.713562, -54.727596, -48.92349, -54.789635, -67.37843, -76.66096, -73.1671, -87.65806, -99.33467, -104.658676, -105.87637, -114.53355, -115.5239, -125.89807, -139.082, -143.63538, -142.29962, -137.4082, -161.7046, -162.24754, -158.44301, -177.06168, -166.37965, -182.70645, -185.09727, -189.93726, -177.63068, -191.02654, -190.93294, -187.85068, -199.92258, -198.63461, -199.58131, -212.48468, -206.23601, -211.4227, -218.63359, -224.79636, -231.376, -223.78336, -221.19205, -238.71568, -224.2388, -218.01895, -227.49657, -221.69603, -230.26488, -218.36143, -220.43254, -226.64919, -212.59207, -225.32123, -220.1036, -218.30737, -212.10869, -212.29033, -219.89949, -217.26492, -209.3771, -194.17052, -208.0605, -207.79724, -190.80663, -196.26205, -179.92268, -177.2375, -180.13649, -174.19185, -185.63557, -159.33908, -177.71075, -156.08044, -160.24042, -149.11995, -148.48769, -145.0306, -141.22212, -132.08865, -130.66814, -115.70701, -110.78786, -111.53611, -88.06789, -85.0113, -82.30008, -80.4348, -63.297966, -67.03102, -70.61455, -56.25191, -48.426514, -54.862167, -24.250004, -27.4897, -20.009115, -15.960924, -3.9002838, -3.0750127, 7.9596715, 11.897266, 18.190056, 17.879662, 29.245876, 46.287605, 53.375774, 46.94959, 54.422523, 60.666332, 72.03676, 88.16187, 90.36747, 102.50478, 108.757454, 97.650986, 99.188896, 114.70395, 122.728615, 132.6987, 137.99367, 132.7435, 153.39764, 147.1321, 164.48956, 163.52798, 170.3947, 168.1754, 172.3494, 169.42416, 184.68484, 190.67664, 202.68398, 189.91632, 198.7794, 180.81807, 205.98648, 201.85915, 200.43373, 206.5106, 219.85347, 208.69815, 209.30867, 223.7762, 220.72722, 223.2816, 227.40543, 228.72081, 219.78961, 230.52316, 214.70453, 228.9469, 226.88087, 220.47495, 226.35178, 216.19508, 224.42451, 231.71278, 221.00325, 219.58595, 217.02516, 220.29698, 208.59154, 214.44919, 203.6927, 204.59872, 198.27487, 208.59032, 196.07826, 182.98662, 194.0817, 197.29701, 183.16739, 176.6386, 169.10585, 168.02623, 159.49901, 167.34134, 145.68178, 152.82971, 155.92667, 137.73132, 125.37648, 121.95651, 130.35976, 109.6605, 104.22374, 99.8873, 93.73692, 81.82534, 85.39096, 77.29339, 76.9015, 61.32132, 63.058514, 47.099796, 50.954193, 50.66741, 38.586464, 32.628365, 20.243225, -0.543707, 1.3718911, -9.965812, -4.918854, -20.659986, -21.29536, -35.024624, -26.80005, -50.65987, -60.02072, -64.856705, -64.614235, -64.47722, -83.000854, -89.89356, -78.78776, -95.82681, -112.40337, -105.334435, -124.30159, -114.20824, -137.17639, -145.09247, -140.6235, -152.53023, -136.4462, -153.59256, -153.75804, -168.29639, -166.5256, -170.57632, -182.87956, -182.04213, -180.40059, -177.81673, -193.39775, -198.54865, -207.83261, -202.89453, -207.00389, -211.68834, -216.36166, -221.04611, -216.63249, -222.57925, -219.53767, -230.2445, -224.17224, -231.32968, -221.70856, -223.50304, -235.28732, -222.19725, -220.36324, -230.63898, -220.74786, -219.46996, -230.087, -234.26997, -213.71347, -219.00986, -226.50276, -209.39343, -213.43108, -211.96289, -211.9526, -216.1907, -209.97124, -209.4958, -211.62073, -188.33899, -192.90564, -197.08469, -197.38191, -201.43564, -191.82063, -178.10408, -175.50491, -175.76686, -162.80537, -161.03969, -153.20654, -145.52484, -138.44797, -140.97295, -122.498276, -122.924255, -128.52802, -120.87051, -99.88957, -113.64146, -98.56741, -83.609566, -73.55968, -71.48554, -62.634636, -72.56406, -51.31056, -41.018757, -44.5892, -38.850246, -27.694149, -27.45748, -14.031494, -9.012678, 3.604988, 10.385417, 11.04624, 19.269693, 24.92719, 31.908287, 43.763462, 52.73765, 61.4191, 56.877792, 63.771236, 78.75281, 72.478195, 90.39417, 88.109146, 96.543846, 100.78109, 96.01131, 117.468925, 131.65454, 129.93428, 142.07764, 140.33061, 146.68456, 148.4432, 158.57275, 160.6325, 162.39287, 161.7471, 180.93785, 178.53804, 182.34018, 185.196, 200.07242, 192.70438, 194.67729, 210.2352, 211.40404, 216.55977, 212.91757, 211.78537, 217.2809, 219.96043, 229.75339, 226.95532, 227.97797, 222.12889, 233.0053, 223.70537, 228.38742, 216.95148, 240.15051, 221.6748, 231.67809, 236.27399, 230.73564, 222.9632, 212.42694, 218.36899, 224.21104, 222.28925, 225.41986, 216.4955, 213.7453, 205.40315, 209.40215, 214.2659, 192.2181, 210.69362, 191.06436, 199.70534, 199.02957, 189.33354, 193.68567, 166.20355, 182.53204, 171.92102, 168.01964, 167.3507, 154.99086, 156.5526, 144.41571, 132.90125, 135.5564, 134.13127, 125.323265, 116.47573, 117.312546, 113.30317, 105.49649, 88.9999, 81.25897, 80.16432, 79.0299, 63.06093, 59.414402, 57.270725, 43.2651, 34.847187, 29.618114, 19.437489, 7.0658827, 7.600524, 6.9791007, 5.6758156, -24.94667, -16.21037, -18.972443, -35.06812, -31.659647, -58.977955, -51.308926, -63.739487, -52.388584, -75.53302, -86.96514, -86.54274, -94.37706, -95.75903, -98.93723, -122.98011, -119.11197, -129.43541, -137.72845, -132.60059, -144.76172, -129.41695, -141.30032, -149.16454, -165.61288, -160.94592, -180.72523, -178.04205, -175.07417, -185.70932, -194.9487, -215.27516, -204.8794, -198.27405, -203.27026, -210.9389, -210.79875, -211.41823, -216.92145, -226.76741, -228.09259, -226.59863, -226.93384, -218.58965, -232.6621, -227.31999, -223.76617, -222.95996, -237.87843, -230.08827, -242.28506, -233.20161, -236.04778, -248.10454, -227.3035, -221.78525, -234.02606, -234.57439, -228.39024, -232.71724, -213.87296, -218.61226, -214.93523, -215.5322, -216.28143, -200.43129, -204.58078, -200.21907, -192.10545, -191.75145, -191.92252, -193.58922, -179.6754, -176.72122, -184.62015, -171.99701, -172.70607, -156.19345, -149.43349, -161.16727, -144.92839, -135.78494, -126.503204, -133.8875, -144.13606, -108.27872, -116.4196, -104.24913, -90.74542, -102.44169, -78.29863, -70.07097, -73.7078, -54.19364, -60.67234, -67.25464, -42.435074, -34.2886, -30.314848, -13.145017, -20.01361, -4.21594, 0.064736515, 2.4084709, 19.219986, 30.498182, 18.53273, 39.15228, 45.051594, 55.515266, 60.52198, 60.178104, 67.61151, 85.70726, 92.37867, 89.25301, 91.222885, 91.51169, 101.93133, 120.37886, 121.949486, 125.6729, 137.65681, 141.2113, 151.1532, 157.71944, 161.16461, 166.42212, 166.95401, 171.33864, 164.29048, 173.43152, 178.34148, 170.35924, 179.11931, 200.8255, 197.54456, 196.47092, 206.18446, 208.19757, 213.39809, 213.32782, 217.56464, 214.76566, 223.96092, 226.30348, 217.53354, 226.09027, 227.06355, 228.33377, 224.4155, 232.40291, 227.15439, 233.65532, 248.98943, 240.16502, 239.6272, 229.76744, 233.22995, 233.43077, 241.12576, 220.00548, 222.76698, 227.86163, 224.71399, 223.29001, 224.38144, 228.60452, 210.81876, 201.94919, 207.59448, 197.21153, 209.4182, 188.88947, 189.98544, 194.7179, 176.36284, 180.80763, 181.88676, 181.27258, 169.33414, 156.19315, 147.8148, 149.71138, 139.86942, 136.81906, 134.42563, 121.170746, 121.980415, 103.93431, 117.83953, 110.1181, 92.10058, 84.75976, 85.38461, 72.98432, 69.81224, 72.04351, 61.270367, 49.615128, 39.208076, 38.006233, 29.152119, 23.36454, 14.37649, 5.9464965, -6.059558, -2.919202, -12.013117, -26.31435, -30.9535, -46.050182, -33.190845, -43.503426, -55.06196, -56.88122, -63.11981, -80.56166, -88.7032, -94.04254, -101.254745, -105.85316, -116.92842, -116.22277, -116.84191, -125.20928, -137.22263, -130.16248, -148.58324, -155.17738, -151.13214, -167.15578, -174.65527, -183.39417, -169.45216, -189.73381, -194.52983, -181.30653, -201.89906, -180.01807, -191.3532, -186.62784, -199.41393, -214.4084, -226.20038, -224.53294, -218.81161, -230.30963, -223.38037, -232.37938, -230.28305, -230.51686, -241.7858, -239.01065, -227.41351, -241.16652, -216.11618, -237.19186, -240.20108, -234.55403, -247.92758, -227.45413, -231.249, -241.78831, -241.78073, -224.05835, -221.67828, -226.58203, -224.8204, -231.93288, -211.77267, -214.59178, -210.78539, -222.91719, -214.9175, -202.27892, -195.6235, -196.707, -194.71265, -195.57259, -199.6146, -171.22546, -175.16553, -165.4787, -170.11821, -167.69803, -145.75528, -154.57838, -150.63283, -131.8153, -138.59885, -130.00133, -129.90685, -130.9601, -113.59628, -108.70955, -95.99347, -86.45991, -77.10719, -74.11912, -73.27584, -68.13497, -59.12619, -37.171383, -41.11133, -28.751776, -27.456259, -22.591515, -12.58267, -2.3062742, 7.1039014, 5.05771, 21.769709, 17.953651, 37.266964, 46.98801, 34.706673, 53.620975, 62.053497, 54.506416, 75.196, 78.294106, 90.4567, 103.15029, 101.33899, 111.59946, 103.172585, 117.13067, 119.31266, 125.85138, 126.218864, 146.90509, 143.07071, 145.20027, 160.21939, 157.24147, 170.45576, 174.78131, 167.68028, 188.37741, 186.8264, 190.88898, 195.32193, 199.62619, 202.2171, 210.66972, 205.2362, 217.24638, 215.0903, 228.17322, 229.34854, 227.31358, 238.49039, 236.40921, 237.59517, 232.756, 233.17802, 239.65971, 240.11176, 243.38127, 238.59631, 240.28441, 229.68417, 240.92986, 224.87207, 233.78537, 221.22559, 228.18613, 240.32063, 235.6941, 231.71169, 223.74525, 226.43544, 235.75893, 219.89467, 225.58168, 222.37663, 214.89958, 206.69623, 207.45984, 208.4675, 201.71025, 189.69707, 193.8702, 189.31927, 181.17403, 186.14241, 162.59264, 176.19717, 161.10255, 159.03432, 148.25844, 142.21342, 135.98094, 135.46321, 129.9887, 121.125, 119.359825, 112.96096, 99.75066, 100.87692, 87.79043, 75.423416, 76.5103, 71.91428, 53.39801, 60.211464, 61.59947, 46.95931, 41.14079, 20.690647, 28.057049, 25.005003, 4.6531277, -3.9015381, -5.959566, -11.490997, -22.900303, -37.363914, -46.984818, -41.25932, -45.264133, -61.81599, -58.56495, -71.720085, -84.25696, -85.264114, -91.36501, -97.86247, -119.30839, -105.80542, -112.82759, -131.85, -136.08983, -126.90728, -161.5913, -154.3644, -156.21477, -154.22754, -175.86066, -168.4935, -176.12051, -184.59334, -186.97075, -190.59789, -190.69078, -202.03844, -210.24371, -210.36417, -216.05205, -216.78864, -219.5597, -218.99648, -218.54895, -218.5645, -226.83875, -223.84291, -230.10704, -225.85123, -243.239, -244.06252, -240.92868, -245.38756, -242.94891, -247.97195, -249.57152, -245.69287, -238.29909, -240.57254, -243.75761, -248.15286, -231.31349, -229.72934, -233.18274, -236.42204, -225.53929, -239.02425, -225.29993, -220.73122, -222.74014, -213.95844, -225.09038, -201.66656, -208.59552, -218.67822, -197.5203, -182.75623, -194.4341, -184.64923, -194.42119, -178.87265, -175.2033, -157.66473, -151.95383, -158.82819, -145.29083, -147.76532, -150.9155, -136.0943, -124.48386, -119.559494, -110.194496, -111.114395, -99.294495, -110.929535, -77.404144, -90.80548, -69.076706, -61.99092, -58.731777, -62.216713, -48.561085, -42.444077, -41.64907, -19.57523, -17.18393, -18.030684, -0.28930485, -8.861638, 11.80865, 21.378145, 29.932846, 37.682457, 42.190994, 41.321423, 59.414005, 62.18999, 56.334892, 70.90938, 84.8603, 82.87171, 94.27547, 105.75505, 104.89313, 112.34328, 118.05685, 128.87437, 140.20222, 138.4945, 145.37732, 160.60907, 171.222, 162.98419, 176.97598, 180.81065, 165.8446, 173.11644, 191.04437, 194.35542, 196.15111, 195.83359, 205.9814, 210.19788, 217.28749, 227.20012, 222.5102, 217.28685, 229.80743, 235.56027, 230.26237, 231.89746, 234.08266, 237.54907, 247.80429, 248.03885, 255.39517, 233.9268, 247.98766, 255.47662, 252.37535, 247.93785, 248.97832, 248.58961, 242.48552, 248.04869, 247.33606, 241.19934, 235.83276, 236.9803, 232.87915, 235.24355, 234.36829, 228.95796, 226.07254, 228.11215, 210.34186, 213.25417, 214.92537, 196.32349, 206.47372, 200.60936, 202.57101, 195.69235, 181.65184, 181.85254, 171.46072, 176.49141, 168.42769, 157.30757, 159.85437, 143.68604, 138.2115, 145.21106, 126.55622, 119.84155, 115.18482, 114.2919, 114.5811, 90.93753, 96.940094, 88.39264, 69.73761, 62.242447, 58.253178, 54.98118, 57.545948, 37.61859, 44.700275, 23.389826, 18.180378, 8.788568, 7.63111, -2.3408031, -20.35684, -31.904673, -29.736116, -45.362446, -39.731987, -48.338234, -59.64815, -68.355255, -71.450264, -74.80523, -69.33154, -99.98338, -99.99154, -110.86859, -107.6898, -133.08688, -131.41586, -136.79744, -138.40483, -140.13982, -148.28847, -144.14781, -166.96478, -168.94572, -157.32263, -180.55943, -183.74432, -183.56038, -204.44196, -187.8401, -203.16223, -200.36534, -214.28946, -217.60773, -226.15976, -226.79547, -215.7686, -233.73387, -221.88524, -238.5837, -230.3066, -237.2343, -239.96379, -258.51648, -244.98116, -245.8142, -238.92058, -255.80595, -259.80142, -246.25043, -247.0839, -251.66496, -248.43178, -247.22472, -256.47433, -255.29813, -239.96552, -247.01314, -254.88095, -232.43222, -250.52255, -243.10936, -241.74316, -244.05882, -225.61313, -222.97368, -231.03333, -217.85245, -217.28844, -211.12088, -215.52019, -194.54953, -198.45088, -185.38731, -195.20348, -189.24843, -179.72389, -178.9229, -159.69756, -167.09644, -165.49525, -167.21753, -153.35828, -143.01315, -122.60425, -121.09726, -111.623215, -109.297195, -106.20199, -98.41947, -101.19054, -73.12552, -73.146416, -72.47287, -51.850876, -60.675674, -40.74345, -46.31597, -27.07335, -22.389273, -15.012141, -7.138585, 9.442156, 5.560839, 12.655911, 20.788174, 31.795942, 30.247482, 57.405148, 58.66045, 70.9677, 79.88132, 82.462776, 82.8082, 91.98801, 97.44426, 105.59329, 101.45587, 110.180145, 127.85169, 128.27898, 134.30516, 146.51244, 148.23737, 158.0008, 168.70413, 170.96338, 167.80357, 186.14026, 180.7771, 184.64178, 200.38069, 201.42645, 188.60065, 206.2803, 203.11288, 211.7788, 217.69536, 237.79037, 229.65442, 228.31454, 220.99568, 226.2144, 232.33264, 226.924, 244.77922, 240.5005, 239.85294, 247.37993, 246.76561, 248.19731, 251.01076, 250.99915, 260.0457, 257.34433, 250.12717, 256.22098, 252.77235, 244.72252, 242.3681, 234.68697, 253.29652, 258.43564, 259.8983, 241.60231, 238.73944, 230.90057, 221.58528], [-192.24, -195.84, -199.2, -202.31999, -205.20001, -207.84, -210.48, -212.88, -215.04001, -216.95999, -218.64, -220.31999, -221.76001, -222.72, -223.68, -224.4, -225.12001, -225.36, -225.6, -225.36, -225.12001, -224.64, -223.92001, -222.96, -222.0, -220.56001, -219.12, -217.44, -215.52, -213.36, -210.96, -208.56, -205.68, -202.8, -199.68001, -196.56, -192.96, -189.36, -185.76, -181.68001, -177.6, -173.28, -168.72, -164.16, -159.36, -154.56, -149.52, -144.24, -138.95999, -133.44, -127.92, -122.16, -116.4, -110.4, -104.4, -98.4, -92.16, -85.920006, -79.44, -72.96, -66.48, -60.0, -53.28, -46.56, -39.84, -33.12, -26.4, -19.68, -12.72, -6.0, 0.96000004, 7.6800003, 14.64, 21.36, 28.08, 35.04, 41.76, 48.480003, 54.96, 61.68, 68.16, 74.64, 81.12, 87.600006, 93.840004, 99.840004, 106.08, 112.08, 117.84, 123.6, 129.36, 134.87999, 140.4, 145.68, 150.72, 155.76, 160.56001, 165.36, 169.92, 174.48, 178.56, 182.64, 186.72, 190.31999, 193.92001, 197.28, 200.64, 203.76, 206.40001, 209.04, 211.68001, 213.84, 216.0, 217.92, 219.6, 221.04001, 222.24, 223.2, 224.16, 224.87999, 225.36, 225.36, 225.6, 225.36, 224.87999, 224.4, 223.44, 222.48, 221.28, 219.84, 218.40001, 216.48, 214.56, 212.16, 209.76001, 207.12, 204.48, 201.36, 198.23999, 194.87999, 191.28, 187.68001, 183.84, 179.76001, 175.44, 171.12, 166.56, 162.0, 157.2, 152.16, 147.12, 141.84001, 136.32, 130.8, 125.28001, 119.52, 113.52, 107.76, 101.520004, 95.520004, 89.28, 82.8, 76.56, 70.08, 63.36, 56.88, 50.16, 43.44, 36.72, 30.0, 23.28, 16.320002, 9.599999, 2.6399999, -4.0800004, -11.04, -17.76, -24.48, -31.439999, -38.16, -44.88, -51.600002, -58.079998, -64.8, -71.28, -77.76, -84.240005, -90.48, -96.72, -102.72, -108.96, -114.71999, -120.72, -126.48, -132.0, -137.52, -142.8, -148.08, -153.12, -158.15999, -162.96, -167.52, -172.08, -176.40001, -180.48, -184.56, -188.40001, -192.24, -195.6, -198.95999, -202.08, -204.95999, -207.84, -210.23999, -212.64, -214.79999, -216.95999, -218.64, -220.31999, -221.51999, -222.72, -223.68, -224.4, -225.12001, -225.36, -225.6, -225.36, -225.12001, -224.64, -223.92001, -223.2, -222.0, -220.8, -219.12, -217.44, -215.52, -213.36, -211.2, -208.56, -205.92, -203.04001, -199.92, -196.8, -193.2, -189.6, -185.76, -181.92, -177.84, -173.52, -168.95999, -164.4, -159.6, -154.79999, -149.76001, -144.48, -139.2, -133.68, -128.15999, -122.63999, -116.64, -110.880005, -104.880005, -98.64, -92.399994, -86.159996, -79.92, -73.44, -66.96001, -60.239998, -53.760002, -47.039997, -40.32, -33.6, -26.880001, -19.92, -13.2, -6.2400002, 0.48000002, 7.44, 14.16, 20.88, 27.84, 34.559998, 41.280003, 48.0, 54.72, 61.199997, 67.92, 74.4, 80.880005, 87.12, 93.36, 99.6, 105.6, 111.6, 117.600006, 123.36, 129.12, 134.64, 139.92, 145.20001, 150.48, 155.52, 160.31999, 165.12001, 169.68001, 174.24, 178.31999, 182.4, 186.48, 190.31999, 193.68, 197.28, 200.4, 203.52, 206.40001, 209.04, 211.44, 213.84, 215.76, 217.68001, 219.36, 220.8, 222.24, 223.2, 224.16, 224.87999, 225.12001, 225.36, 225.6, 225.36, 224.87999, 224.4, 223.68, 222.48, 221.28, 220.08, 218.40001, 216.48, 214.56, 212.4, 210.0, 207.36, 204.48, 201.59999, 198.48001, 195.12001, 191.51999, 187.92, 184.08, 180.0, 175.68, 171.36, 166.8, 162.24, 157.44, 152.4, 147.36, 142.08, 136.56, 131.28, 125.520004, 119.76, 114.0, 108.0, 102.0, 95.759995, 89.52, 83.28, 76.799995, 70.32, 63.84, 57.120003, 50.64, 43.92, 37.2, 30.480001, 23.519999, 16.8, 10.08, 3.1200001, -3.8400002, -10.559999, -17.279999, -24.240002, -30.96, -37.68, -44.4, -51.12, -57.84, -64.32, -71.04, -77.28, -83.76, -90.0, -96.24, -102.479996, -108.479996, -114.479996, -120.24, -125.99999, -131.76001, -137.04, -142.56, -147.84, -152.88, -157.92, -162.72, -167.28, -171.84001, -176.16, -180.23999, -184.32, -188.15999, -192.0, -195.36, -198.72, -201.84001, -204.95999, -207.6, -210.23999, -212.64, -214.79999, -216.72, -218.64, -220.08, -221.51999, -222.72, -223.68, -224.4, -225.12001, -225.36, -225.6, -225.36, -225.12001, -224.64, -223.92001, -223.2, -222.0, -220.8, -219.36, -217.68001, -215.76, -213.59999, -211.2, -208.8, -206.16, -203.28, -200.16, -196.8, -193.44, -189.84, -186.0, -182.16, -178.08, -173.76, -169.2, -164.64, -160.08, -155.04001, -150.0, -144.95999, -139.43999, -134.16, -128.64, -122.880005, -117.12, -111.12, -105.119995, -99.119995, -92.88, -86.64, -80.159996, -73.68, -67.2, -60.719997, -54.0, -47.52, -40.8, -34.08, -27.119999, -20.4, -13.68, -6.7200003, 0.0, 6.96, 13.68, 20.640001, 27.36, 34.08, 41.04, 47.760002, 54.239998, 60.960003, 67.439995, 73.92, 80.4, 86.88, 93.12, 99.119995, 105.36, 111.36, 117.12, 123.12, 128.64, 134.16, 139.68001, 144.95999, 150.23999, 155.28, 160.08, 164.87999, 169.43999, 174.0, 178.08, 182.16, 186.24, 190.08, 193.68, 197.04, 200.16, 203.28, 206.16, 208.8, 211.44, 213.59999, 215.76, 217.68001, 219.36, 220.8, 222.0, 223.2, 224.16, 224.64, 225.12001, 225.36, 225.6, 225.36, 224.87999, 224.4, 223.68, 222.72, 221.51999, 220.08, 218.40001, 216.72, 214.79999, 212.4, 210.0, 207.6, 204.72, 201.84001, 198.72, 195.36, 191.76001, 188.15999, 184.32, 180.23999, 175.92, 171.59999, 167.28, 162.48, 157.68001, 152.64, 147.6, 142.31999, 137.04, 131.51999, 125.759995, 120.24, 114.240005, 108.24, 102.24, 96.24, 90.0, 83.52, 77.28, 70.799995, 64.32, 57.6, 50.88, 44.4, 37.440002, 30.720001, 24.0, 17.279999, 10.320001, 3.6, -3.3600001, -10.08, -17.04, -23.76, -30.720001, -37.440002, -44.16, -50.88, -57.359997, -64.079994, -70.56, -77.04, -83.52, -89.76, -96.0, -102.24, -108.24, -114.240005, -120.0, -125.759995, -131.28, -136.8, -142.31999, -147.36, -152.64, -157.44, -162.48, -167.04, -171.59999, -175.92, -180.0, -184.08, -187.92, -191.76001, -195.12001, -198.48001, -201.59999, -204.72, -207.36, -210.0, -212.4, -214.56, -216.72, -218.40001, -220.08, -221.51999, -222.72, -223.68, -224.4, -224.87999, -225.36, -225.6, -225.36, -225.12001, -224.64, -224.16, -223.2, -222.24, -220.8, -219.36, -217.68001, -215.76, -213.59999, -211.44, -209.04, -206.16, -203.28, -200.4, -197.04, -193.68, -190.08, -186.24, -182.4, -178.31999, -174.0, -169.68001, -164.87999, -160.31999, -155.28, -150.23999, -145.20001, -139.92, -134.4, -128.88, -123.12, -117.36, -111.6, -105.6, -99.36, -93.12, -86.88, -80.64, -74.159996, -67.68, -61.199997, -54.48, -47.760002, -41.04, -34.32, -27.6, -20.88, -13.92, -7.2, -0.24000001, 6.48, 13.440001, 20.16, 27.119999, 33.84, 40.56, 47.28, 54.0, 60.48, 67.2, 73.68, 80.159996, 86.4, 92.64, 98.88, 104.880005, 110.880005, 116.88, 122.63999, 128.40001, 133.92001, 139.43999, 144.72, 150.0, 155.04001, 159.84, 164.64, 169.2, 173.52, 177.84, 182.16, 186.0, 189.84, 193.44, 196.8, 200.16, 203.04001, 205.92, 208.8, 211.2, 213.59999, 215.52, 217.44, 219.12, 220.8, 222.0, 223.2, 223.92001, 224.64, 225.12001, 225.36, 225.6, 225.36, 225.12001, 224.4, 223.68, 222.72, 221.51999, 220.08, 218.64, 216.72, 214.79999, 212.64, 210.23999, 207.6, 204.95999, 202.08, 198.72, 195.6, 192.0, 188.40001, 184.56, 180.48, 176.40001, 171.84001, 167.52, 162.72, 157.92, 152.88, 147.84, 142.56, 137.28, 131.76001, 126.240005, 120.479996, 114.71999, 108.72, 102.72, 96.48, 90.24, 84.0, 77.520004, 71.04, 64.56, 58.079998, 51.36, 44.64, 37.920002, 31.199999, 24.48, 17.52, 10.8, 3.8400002, -2.88, -9.84, -16.56, -23.519999, -30.24, -36.96, -43.68, -50.399998, -57.120003, -63.6, -70.08, -76.56, -83.03999, -89.28, -95.520004, -101.76, -107.76, -113.76, -119.76, -125.28001, -131.04001, -136.56, -141.84001, -147.12, -152.4, -157.2, -162.0, -166.8, -171.36, -175.68, -180.0, -183.84, -187.92, -191.51999, -195.12001, -198.48001, -201.59999, -204.48, -207.36, -210.0, -212.4, -214.56, -216.48, -218.40001, -219.84, -221.28, -222.48, -223.68, -224.4, -224.87999, -225.36, -225.6, -225.36, -225.12001, -224.87999, -224.16, -223.2, -222.24, -221.04001, -219.36, -217.68001, -216.0, -213.84, -211.44, -209.04, -206.40001, -203.52, -200.4, -197.28, -193.92001, -190.31999, -186.48, -182.64, -178.56, -174.24, -169.92, -165.36, -160.56001, -155.52, -150.72, -145.44, -140.16, -134.64, -129.12, -123.6, -117.84, -111.84, -105.840004, -99.840004, -93.6, -87.36, -80.880005, -74.64, -67.92, -61.440002, -54.96, -48.24, -41.519997, -34.8, -28.08, -21.119999, -14.4, -7.44, -0.72, 6.2400002, 12.96, 19.92, 26.64, 33.36, 40.079998, 46.8, 53.52, 60.239998, 66.72, 73.200005, 79.68, 86.159996, 92.399994, 98.64, 104.64, 110.64, 116.64, 122.399994, 128.15999, 133.68, 139.2, 144.48, 149.52, 154.56, 159.6, 164.4, 168.95999, 173.28, 177.6, 181.92, 185.76, 189.6, 193.2, 196.56, 199.92, 203.04001, 205.92, 208.56, 210.96, 213.36, 215.52, 217.44, 219.12, 220.56001, 222.0, 222.96, 223.92001, 224.64, 225.12001, 225.36, 225.6, 225.36, 225.12001, 224.4, 223.68, 222.72, 221.51999, 220.31999, 218.64, 216.95999, 215.04001, 212.88, 210.48, 207.84, 205.20001, 202.08, 198.95999, 195.6, 192.24, 188.64, 184.79999, 180.72, 176.64, 172.08, 167.76, 162.96, 158.15999, 153.36, 148.08, 143.04001, 137.52, 132.24, 126.48, 120.72, 114.96, 108.96, 102.96, 96.96001, 90.72, 84.240005, 78.0, 71.520004, 65.04, 58.32, 51.84, 45.12, 38.399998, 31.68, 24.72, 18.0, 11.04, 4.3199997, -2.6399999, -9.360001, -16.320002, -23.04, -29.76, -36.48, -43.44, -49.920002, -56.64, -63.36, -69.840004, -76.32, -82.8, -89.04, -95.28001, -101.520004, -107.520004, -113.52, -119.28, -125.04001, -130.8, -136.32, -141.59999, -146.88, -151.92, -156.95999, -161.76001, -166.56, -171.12, -175.44, -179.76001, -183.59999, -187.68001, -191.28, -194.87999, -198.23999, -201.36, -204.24, -207.12, -209.76001, -212.16, -214.32, -216.48, -218.15999, -219.84, -221.28, -222.48, -223.44, -224.4, -224.87999, -225.36, -225.6, -225.36, -225.36, -224.87999, -224.16, -223.2, -222.24, -221.04001, -219.6, -217.92, -216.0, -213.84, -211.68001, -209.28, -206.64, -203.76, -200.64, -197.52, -194.16, -190.56001, -186.72, -182.88, -178.8, -174.48, -170.16, -165.6, -160.8, -156.0, -150.96, -145.68, -140.4, -135.12001, -129.6, -123.84, -118.08, -112.08, -106.08, -100.08, -93.840004, -87.600006, -81.36, -74.880005, -68.4, -61.92, -55.2, -48.480003, -42.0, -52.559998, -42.48, -32.4, -22.08, -11.759999, -1.6800001, 8.639999, 18.960001, 29.039999, 39.36, 49.44, 59.52, 69.6, 79.68, 89.52, 99.36, 108.96, 118.8, 128.15999, 137.76, 146.88, 156.0, 165.12001, 174.0, 182.64, 191.28, 199.43999, 207.6, 215.76, 223.44, 231.12, 238.31999, 245.52, 252.48001, 259.2, 265.68, 271.68, 277.68, 283.44, 288.96, 294.0, 299.04, 303.6, 307.91998, 312.0, 315.6, 319.2, 322.32, 325.2, 327.84003, 330.24002, 332.15997, 333.84, 335.28, 336.24, 336.96002, 337.44, 337.68, 337.44, 336.96002, 336.0, 335.04, 333.6, 331.92, 329.75998, 327.36, 324.72, 321.84, 318.72, 315.12, 311.28, 307.19998, 302.88, 298.08, 293.28, 288.0, 282.48, 276.72, 270.72, 264.48, 258.0, 251.28001, 244.56001, 237.36, 229.92, 222.24, 214.56, 206.40001, 198.23999, 189.84, 181.2, 172.56, 163.68, 154.56, 145.44, 136.07999, 126.72, 117.12, 107.520004, 97.68, 87.84, 78.0, 67.92, 57.84, 47.760002, 37.68, 27.6, 17.279999, 6.96, -3.1200001, -13.440001, -23.76, -33.84, -44.16, -54.239998, -64.32, -74.4, -84.240005, -94.079994, -103.92, -113.52, -123.12, -132.72, -142.08, -151.2, -160.31999, -169.2, -178.08, -186.72, -195.12001, -203.52, -211.44, -219.36, -227.04, -234.48, -241.92, -248.87999, -255.6, -262.32, -268.56, -274.56, -280.56, -286.08002, -291.36, -296.4, -301.2, -305.52, -309.84, -313.68002, -317.28, -320.63998, -323.76, -326.63998, -329.04, -331.2, -332.88, -334.56, -335.76, -336.72, -337.19998, -337.44, -337.44, -337.19998, -336.47998, -335.52, -334.32, -332.88, -330.96, -328.8, -326.16, -323.52002, -320.40002, -317.04, -313.44, -309.36002, -305.28, -300.72, -295.92, -290.88, -285.6, -279.84, -274.08, -267.84003, -261.6, -254.88, -248.16, -241.2, -233.76, -226.32, -218.64, -210.72, -202.56, -194.4, -185.76, -177.12, -168.48001, -159.36, -150.48, -141.12, -131.76001, -122.16, -112.560005, -102.96, -93.12, -83.28, -73.200005, -63.36, -53.28, -42.960003, -32.879997, -22.56, -12.4800005, -2.1599998, 8.160001, 18.24, 28.560001, 38.64, 48.96, 59.04, 69.119995, 78.96, 89.04, 98.88, 108.479996, 118.08, 127.68, 137.04, 146.40001, 155.52, 164.64, 173.52, 182.16, 190.8, 198.95999, 207.36, 215.28, 222.96, 230.64, 238.08, 245.04001, 251.99998, 258.72, 265.2, 271.44, 277.44, 283.19998, 288.48, 293.76, 298.56, 303.36002, 307.68, 311.76, 315.6, 318.96, 322.32, 325.2, 327.6, 330.0, 331.92, 333.6, 335.04, 336.24, 336.96002, 337.44, 337.68, 337.44, 336.96002, 336.24, 335.04, 333.6, 331.92, 330.0, 327.6, 324.96, 322.08002, 318.96, 315.36002, 311.52, 307.44, 303.12, 298.56, 293.52002, 288.24, 282.96, 277.19998, 271.2, 264.96, 258.48, 251.76001, 244.79999, 237.6, 230.4, 222.72, 214.79999, 206.88, 198.72, 190.31999, 181.92, 173.04001, 164.16, 155.28, 145.92, 136.8, 127.2, 117.84, 108.0, 98.4, 88.56, 78.479996, 68.64, 58.56, 48.480003, 38.16, 28.08, 17.76, 7.6800003, -2.6399999, -12.96, -23.04, -33.36, -43.44, -53.52, -63.6, -73.68, -83.76, -93.6, -103.44, -113.03999, -122.63999, -132.24, -141.59999, -150.72, -159.84, -168.72, -177.6, -186.24, -194.64, -203.04001, -210.96, -218.88, -226.56, -234.24, -241.44, -248.4, -255.36, -261.84, -268.08, -274.32, -280.08002, -285.6, -291.12003, -296.16, -300.96, -305.28, -309.59998, -313.44, -317.28, -320.63998, -323.52002, -326.4, -328.8, -330.96, -332.88, -334.32, -335.76, -336.47998, -337.19998, -337.44, -337.44, -337.19998, -336.72, -335.76, -334.32, -332.88, -330.96, -328.8, -326.4, -323.76, -320.63998, -317.28, -313.68002, -309.59998, -305.52, -300.96, -296.16, -291.12003, -285.84, -280.32, -274.32, -268.32, -261.84, -255.36, -248.64, -241.44, -234.24, -226.8, -219.12, -211.2, -203.04001, -194.87999, -186.24, -177.84, -168.95999, -160.08, -150.96, -141.59999, -132.24, -122.880005, -113.28, -103.44, -93.840004, -83.76, -73.92, -63.84, -53.760002, -43.68, -33.36, -23.28, -12.96, -2.88, 7.44, 17.76, 27.84, 38.16, 48.24, 58.32, 68.4, 78.479996, 88.32, 98.16, 108.0, 117.600006, 127.2, 136.56, 145.92, 155.04001, 164.16, 173.04001, 181.68001, 190.31999, 198.48001, 206.88, 214.79999, 222.48, 230.16, 237.6, 244.79999, 251.76001, 258.48, 264.96, 271.2, 276.96002, 282.72, 288.24, 293.52002, 298.32, 303.12, 205.44, 208.08, 210.72, 212.88, 215.04001, 217.2, 218.88, 220.31999, 221.76001, 222.96, 223.92001, 224.64, 225.12001, 225.36, 225.6, 225.36, 225.12001, 224.64, 223.92001, 222.96, 221.76001, 220.56001, 218.88, 217.2, 215.28, 213.12, 210.72, 208.31999, 205.68, 202.56, 199.68001, 196.32, 192.72, 189.12, 185.28, 181.44, 177.36, 173.04001, 168.48001, 163.92001, 159.12, 154.08, 149.04, 143.76, 138.48001, 133.2, 127.44, 121.68001, 115.920006, 110.159996, 103.92, 97.92, 91.68, 85.44, 78.96, 72.479996, 66.0, 59.52, 52.8, 46.32, 39.600002, 32.640003, 25.92, 19.199999, 12.24, 5.52, -1.44, -8.160001, -15.12, -21.84, -28.560001, -35.52, -42.239998, -48.96, -55.440002, -62.16, -68.64, -75.119995, -81.6, -87.84, -94.079994, -100.32, -106.56, -112.32, -118.32, -124.08, -129.84, -135.36, -140.64, -145.92, -151.2, -156.24, -161.04001, -165.6, -170.16, -174.72, -179.04, -183.12, -186.95999, -190.56001, -194.16, -197.52, -200.88, -203.76, -206.64, -209.28, -211.68001, -214.08, -216.0, -217.92, -219.6, -221.04001, -222.24, -223.44, -224.16, -224.87999, -225.36, -225.6, -225.6, -225.36, -224.87999, -224.4, -223.44, -222.48, -221.28, -219.84, -218.15999, -216.24, -214.32, -212.16, -209.76001, -207.12, -204.24, -201.12, -198.0, -194.64, -191.04001, -187.44, -183.59999, -179.52, -175.20001, -170.88, -166.32, -161.51999, -156.72, -151.68001, -146.64, -141.36, -136.07999, -130.56001, -124.799995, -119.04, -113.28, -107.28, -101.28, -95.04, -88.8, -82.32, -76.08, -69.6, -62.879997, -56.4, -49.68, -42.960003, -36.239998, -29.52, -22.8, -15.84, -9.12, -2.1599998, 4.56, 11.52, 18.24, 24.960001, 31.92, 38.64, 45.36, 52.079998, 58.56, 65.28001, 71.76, 78.24, 84.479996, 90.96, 97.2, 103.200005, 109.200005, 115.2, 120.96, 126.72, 132.48, 137.76, 143.28, 148.31999, 153.59999, 158.40001, 163.2, 168.0, 172.31999, 176.64, 180.96, 184.79999, 188.64, 192.48, 195.84, 199.2, 202.31999, 205.20001, 207.84, 210.48, 212.88, 215.04001, 216.95999, 218.64, 220.31999, 221.76001, 222.72, 223.68, 224.64, 225.12001, 225.36, 225.6, 225.36, 225.12001, 224.64, 223.92001, 222.96, 222.0, 220.56001, 219.12, 217.44, 215.52, 213.36, 210.96, 208.56, 205.68, 202.8, 199.68001, 196.56, 192.96, 189.36, 185.52, 181.68001, 177.6, 173.28, 168.72, 164.16, 159.36, 154.32, 149.28, 144.24, 138.95999, 133.44, 127.92, 122.16, 116.4, 110.4, 104.4, 98.16, 92.16, 85.68, 79.44, 72.96, 66.48, 60.0, 53.28, 46.56, 39.84, 33.12, 26.4, 19.44, 12.72, 5.76, -0.96000004, -7.92, -14.64, -21.36, -28.32, -35.04, -41.76, -48.480003, -55.2, -61.68, -68.4, -74.880005, -81.12, -87.600006, -93.840004, -100.08, -106.08, -112.08, -118.08, -123.84, -129.36, -134.87999, -140.4, -145.68, -150.72, -155.76, -160.8, -165.36, -169.92, -174.48, -178.8, -182.88, -186.72, -190.56001, -193.92001, -197.52, -200.64, -203.76, -206.64, -209.28, -211.68001, -213.84, -216.0, -217.92, -219.6, -221.04001, -222.24, -223.2, -224.16, -224.87999, -225.36, -225.36, -225.6, -225.36, -224.87999, -224.4, -223.44, -222.48, -221.28, -219.84, -218.15999, -216.48, -214.32, -212.16, -209.76001, -207.12, -204.48, -201.36, -198.23999, -194.87999, -191.28, -187.68001, -183.84, -179.76001, -175.44, -171.12, -166.56, -162.0, -156.95999, -152.16, -146.88, -141.59999, -136.32, -130.8, -125.04001, -119.52, -113.52, -107.520004, -101.520004, -95.28001, -89.04, -82.8, -76.32, -69.840004, -63.36, -56.88, -50.16, -43.44, -36.72, -30.0, -23.04, -16.320002, -9.599999, -2.6399999, 4.0800004, 11.04, 17.76, 24.72, 31.439999, 38.16, 44.88, 51.600002, 58.32, 64.8, 71.28, 77.76, 84.240005, 90.48, 96.72, 102.96, 108.96, 114.96, 120.72, 126.48, 132.0, 137.52, 142.8, 148.08, 153.12, 158.15999, 162.96, 167.52, 172.08, 176.40001, 180.72, 184.56, 188.40001, 192.24, 195.6, 198.95999, 202.08, 204.95999, 207.84, 210.23999, 212.64, 214.79999, 216.95999, 218.64, 220.31999, 221.51999, 222.72, 223.68, 224.4, 225.12001, 225.36, 225.6, 225.36, 225.12001, 224.64, 223.92001, 223.2, 222.0, 220.56001, 219.12, 217.44, 215.52, 213.36, 211.2, 208.56, 205.92]]
  in  "Stop":bool
  in  "Sample Index":i32=297 min=0 max=499
  in  "Check?":bool
  out "Train Speed (Sample/sec)":dbl=11006.39746853613 format="%#.0g"
  out "Train Speed (sec/iter)":dbl=0.011629599999992024 format="%#.4g"
  out "Train Loss":sgl=6.871157 format="%.3g"
  out "Time_Elapsed":dbl=14.061959599999994 format="%<%H:%M:%S>t"
  out "Session Data":T1={"Epochs"=12.436211, "Tot_Iter"=923, "LR"=5e-05, "LR_iter"=924}
  in  "LR Update Policy":T2={"Policy_Type"=enum."Step", "LR0"=0.0001, "k"=10.0, "WarmUp_Policy"=enum."Ramp", "WarmUp_Iter"=600, "WarmUp_Ratio"=20.0} {"WarmUp_Ratio" min=1; "WarmUp_Iter" min=1; "LR0" format="%.7f"}
  in  "Train_Params":T4={"Optimizer"=enum."Adam", "Beta_1"=0.9, "Beta_2"=0.999, "Weight Decay(L1)"=0.0, "Weight Decay(L2)"=0.0, "Data_Sampling"=enum."Random"}
  in  "NN_Device":T7=enum."GPU"
  # "Waveform Anomaly Detection - Training"
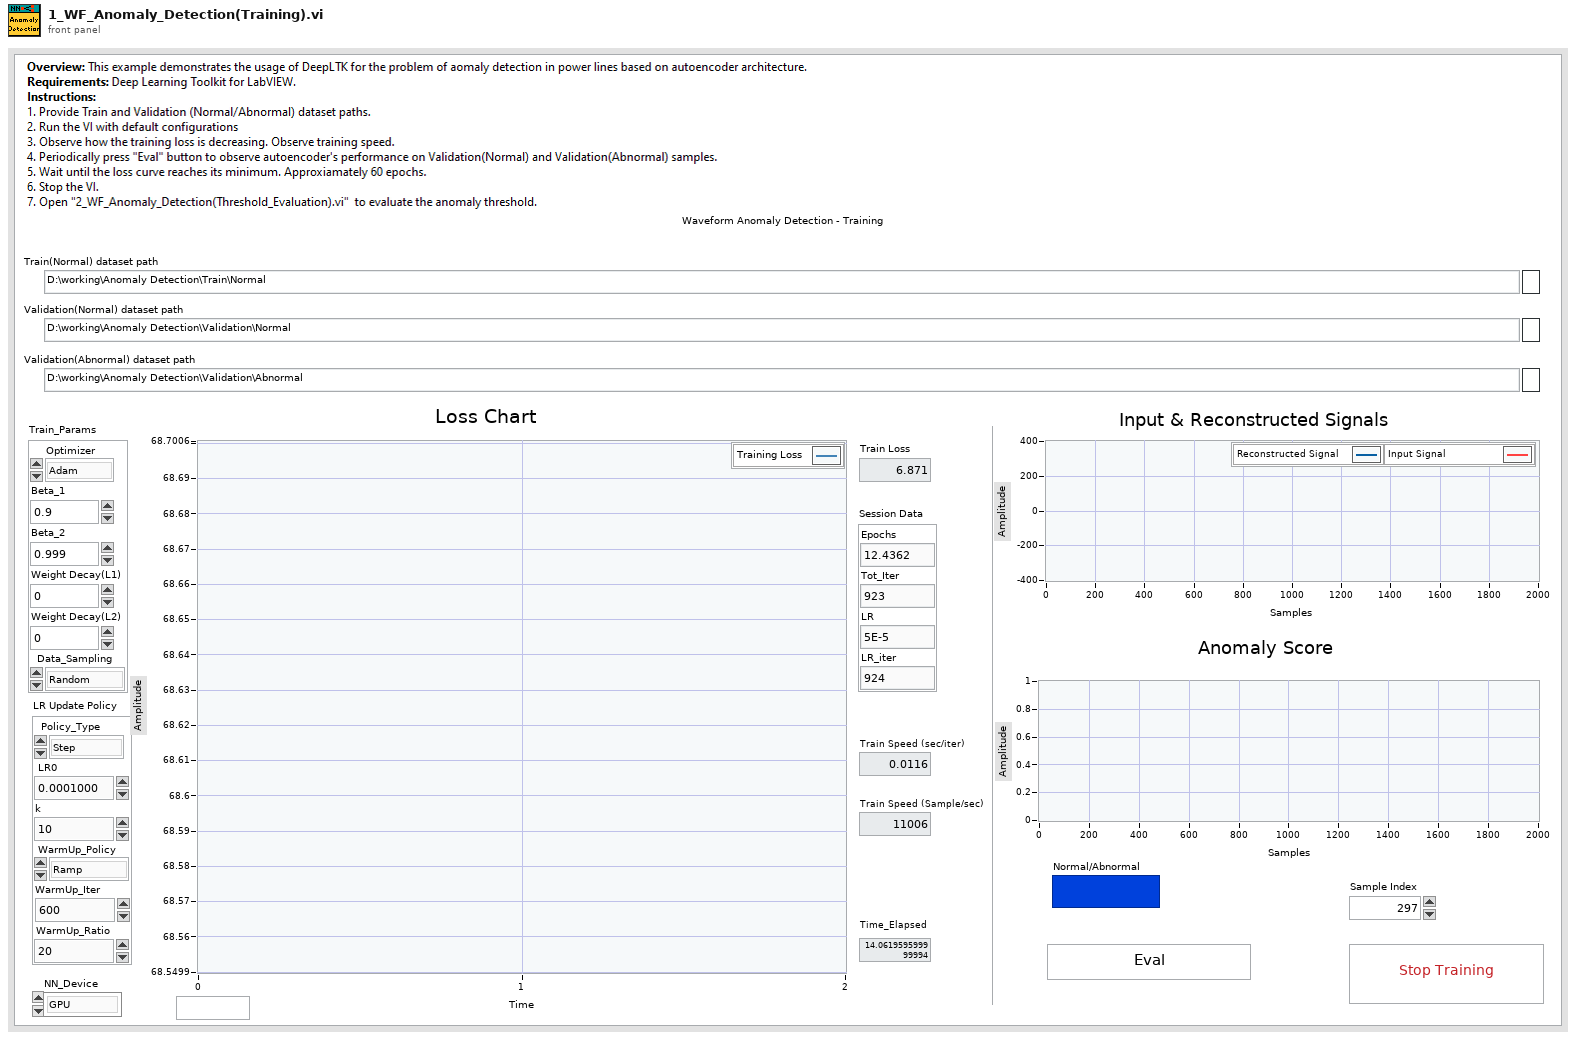
[diagram p1: front panel]
types:
  T1 = typedef "Deep_Learning_Toolkit_by_Ngene.lvlib/NN_Train_Session_Data.ctl" = cluster{"Epochs":sgl, "Tot_Iter":i32, "LR":sgl, "LR_iter":i32}
  T2 = typedef "Deep_Learning_Toolkit_by_Ngene.lvlib/NN_LR_Policy_Cfg.ctl" = cluster{"Policy_Type":T3, "LR0":dbl, "k":sgl, "WarmUp_Policy":enum16{"Step", "Ramp"}, "WarmUp_Iter":i32, "WarmUp_Ratio":sgl}
  T3 = typedef "Deep_Learning_Toolkit_by_Ngene.lvlib/NN_LR_Policy_Type.ctl" = enum16{"Manual", "Step", "Exp", "1/t"}
  T4 = typedef "Deep_Learning_Toolkit_by_Ngene.lvlib/NN_Train_Params.ctl" = cluster{"Optimizer":T5, "Beta_1":sgl, "Beta_2":sgl, "Weight Decay(L1)":sgl, "Weight Decay(L2)":sgl, "Data_Sampling":T6}
  T5 = typedef "Deep_Learning_Toolkit_by_Ngene.lvlib/NN_Train_Optimizer.ctl" = enum16{"SGD", "Adam", "Adagrad", "Adadelta", "RMSProp", "Nesterov"}
  T6 = typedef "Deep_Learning_Toolkit_by_Ngene.lvlib/NN_Train_Data_Sampling.ctl" = enum16{"Random", "Sequential"}
  T7 = typedef "Deep_Learning_Toolkit_by_Ngene.lvlib/NN_Device.ctl" = enum16{"CPU", "GPU"}
  T8 = typedef "Deep_Learning_Toolkit_by_Ngene.lvlib/NN_Layer_Config_Aug(Input1D).ctl" = T9[]
  T9 = typedef "Deep_Learning_Toolkit_by_Ngene.lvlib/NN_Input1D_Aug_Config.ctl" = cluster{"Aug Type(1D)":T10, "Aug Value":sgl, "Distribution":T11}
  T10 = typedef "Deep_Learning_Toolkit_by_Ngene.lvlib/NN_Input1D_Aug_Types.ctl" = enum16{"Add_Noise", "Mult_Noise", "Shift", "Scale"}
  T11 = typedef "Deep_Learning_Toolkit_by_Ngene.lvlib/Aug_Distribution_Type.ctl" = enum16{"Uniform", "Gaussian"}
  T12 = typedef "Deep_Learning_Toolkit_by_Ngene.lvlib/NN_Layer_Config(FC).ctl" = cluster{"Name":string, "Size":i32, "BN":bool, "BN_Params":T13, "Activation":T14, "Has Bias?":bool, "Init_Params":T15, "Custom_Params":string}
  T13 = typedef "Deep_Learning_Toolkit_by_Ngene.lvlib/NN_BN_Params.ctl" = cluster{"epsilon":sgl, "momentum":sgl}
  T14 = typedef "Deep_Learning_Toolkit_by_Ngene.lvlib/NN_Activation_Type.ctl" = enum16{"Sigmoid", "ReLU", "LReLU", "ReLU6", "tanh", "Swish", "Mish", "None"}
  T15 = typedef "Deep_Learning_Toolkit_by_Ngene.lvlib/NN_Layer_Init_Params.ctl" = cluster{"Init_Type":T16, "Value":sgl}
  T16 = typedef "Deep_Learning_Toolkit_by_Ngene.lvlib/NN_Layer_Weight_Init_Type.ctl" = enum16{"Const", "Uniform", "Gaussian", "Xavier"}
  T17 = typedef "Deep_Learning_Toolkit_by_Ngene.lvlib/NN_Layer_Config(Input1D).ctl" = cluster{"Name":string, "Size":i32, "Data_Type":T18, "Shift":sgl, "Scale":sgl}
  T18 = typedef "Deep_Learning_Toolkit_by_Ngene.lvlib/NN_Data_type.ctl" = enum16{"I8", "U8", "I16", "U16", "U32 ARGB", "SGL"}
  T19 = typedef "Deep_Learning_Toolkit_by_Ngene.lvlib/NN_Save_Before_Destroy_Options.ctl" = cluster{"CFG?":bool, "Weights?":bool, "Render?":bool}
  T20 = typedef "Deep_Learning_Toolkit_by_Ngene.lvlib/NN_DataSet(In1D_Out1D).ctl" = cluster{"Inputs Ref.":variant, "Outputs Ref.":T21, "Dims_In":i32, "Dataset_Size":i32, "Dims_Out":i32, "Labels":string[], "File Paths":path[]}
  T21 = typedef "Deep_Learning_Toolkit_by_Ngene.lvlib/NN_Data_ref(2D_SGL).ctl" = refnum<data-value>
  T22 = typedef "Deep_Learning_Toolkit_by_Ngene.lvlib/NN.ctl" = cluster{"Name":string, "No of Layers":i32, "mBatch":i32, "Layers":T23[], "Dimty":T24, "Dims_In":T25, "Dims_Out":T25, "Working_Dir":path, "Train?":bool, "Train_Params":T4, "LR_Update_Policy":T2, "Session Data":T1, "Ground_truth":T26, "NNg_hdls":T27, "NN_Device":T7, "GPU Id":i32, "Labels":string[], "Receptive Field":T28[], "Loss_Type":T29, "Loss_Cfg_Prms":variant, "NNG_WS":T30}
  T23 = typedef "Deep_Learning_Toolkit_by_Ngene.lvlib/NN_Layer_ref.ctl" = refnum<data-value>
  T24 = typedef "Deep_Learning_Toolkit_by_Ngene.lvlib/NN_In_Out_Dim-ty.ctl" = enum8{"In1D_Out1D", "In3D_Out1D", "In3D_Out3D", "In3D_OutBBox"}
  T25 = typedef "Deep_Learning_Toolkit_by_Ngene.lvlib/NN_Dims(C,H,W).ctl" = cluster{"C":i32, "H":i32, "W":i32}
  T26 = typedef "Deep_Learning_Toolkit_by_Ngene.lvlib/NN_Ground_truth.ctl" = cluster{"Y":variant}
  T27 = typedef "Deep_Learning_Toolkit_by_Ngene.lvlib/nng_cuda_handles.ctl" = cluster{"cudnn":u64, "cublas":u64, "stream":u64, "curand":u64}
  T28 = typedef "Deep_Learning_Toolkit_by_Ngene.lvlib/NN_Dims(V,H).ctl" = cluster{"V":i32, "H":i32}
  T29 = typedef "Deep_Learning_Toolkit_by_Ngene.lvlib/NN_Loss_Type.ctl" = enum16{"None", "MSE", "CrossEntropy", "YOLO_v2", "YOLO_v4"}
  T30 = typedef "Deep_Learning_Toolkit_by_Ngene.lvlib/NNG_WS.ctl" = cluster{"NNG_WS_Mem":T31, "Max_WS_Size":i64}
  T31 = typedef "Deep_Learning_Toolkit_by_Ngene.lvlib/NNg_WS_Mem_DVR.ctl" = refnum<data-value>
  T32 = typedef "Deep_Learning_Toolkit_by_Ngene.lvlib/NN_Layer.ctl" = cluster{"Name":string, "Layer_Data":variant, "Layer_Type":T33, "Dims_In":T25, "Layers_In":variant, "Dims_Out":T25, "Layers_Out":variant, "Metrics":T34, "GPU_Data":variant, "mBatch":i32, "NN_Device":T7, "NNg_hdls":T27, "Train?":bool, "Dimty":T35, "RecptField":T36}
  T33 = typedef "Deep_Learning_Toolkit_by_Ngene.lvlib/NN_Layer_Type.ctl" = enum16{"Input1D", "Input3D", "Conv1D", "Conv2D", "Conv2D_Adv", "MaxPool", "AvgPool", "UpSample", "DropOut3D", "ShortCut", "Concat", "SoftMax3D", "FC", "DropOut", "Softmax", "Flatten", "YOLO_v2", "YOLO_v4", "Activation", "BatchNormalization", "Unsupported"}
  T34 = typedef "Deep_Learning_Toolkit_by_Ngene.lvlib/NN_Layer_Metrics.ctl" = cluster{"Data":dbl, "Params":dbl, "Ops":dbl}
  T35 = typedef "Deep_Learning_Toolkit_by_Ngene.lvlib/NN_Layer_Dimty.ctl" = enum16{"1D", "3D"}
  T36 = typedef "Deep_Learning_Toolkit_by_Ngene.lvlib/NN_Layer_RF_State.ctl" = cluster{"Dims":T28, "J":T28}
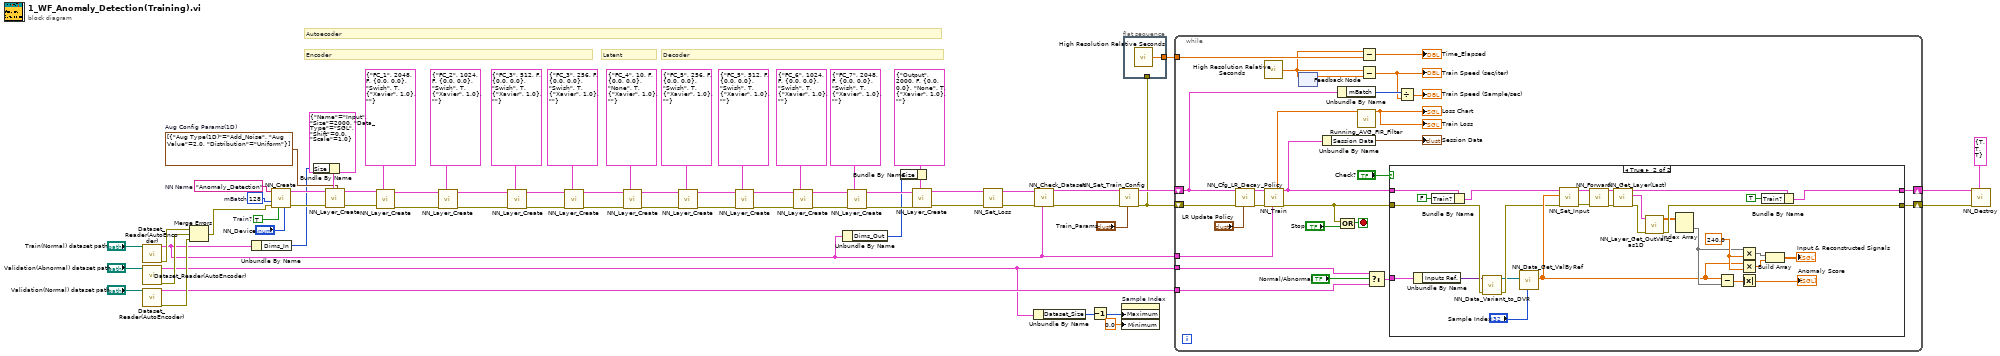
[diagram p0: block diagram]
diagram:
  w17 = T8 [{"Aug Type(1D)"=enum."Add_Noise", "Aug Value"=2.0, "Distribution"=enum."Uniform"}]  # Aug Config Params(1D)
  w59 = TRUE  # Train?
  w63 = 128  # mBatch
  w68 = "Anomaly_Detection"  # NN Name
  # "Latent"
  # "Decoder"
  # "Encoder"
  # "Autoecoder"
  n1 = call "Dataset_Reader(AutoEncoder).vi"("Train dataset path"="Train(Normal) dataset path") -> ("error out"=w6:errorcluster, "Dataset"=w2:T20)  [unwired: 9 in]
  n2 = call "Dataset_Reader(AutoEncoder).vi"("Train dataset path"="Validation(Abnormal) dataset path") -> ("error out"=w7:errorcluster, "Dataset"=w1:T20)  [unwired: 9 in]
  n3 = call "Dataset_Reader(AutoEncoder).vi"("Train dataset path"="Validation(Normal) dataset path") -> ("error out"=w5:errorcluster, "Dataset"=w3:T20)  [unwired: 9 in]
  n4 = Merge Errors(w6, w7, w5) -> (w4:errorcluster)
  n5 = Unbundle By Name(w2) -> ("Dims_In"=w15:i32)
  n6 = call <vilib>:"NN_Create.vi"("NN_Device"="NN_Device", "Train? (false)"=w59, "error in (no error)"=w4, "mBatch (1)"=w63, "Name"=w68) -> ("error out"=w66:errorcluster, "NN out"=w67:T22)  [unwired: 5 in]
  n7 = Bundle By Name(cluster=T17 {"Name"="Input", "Size"=2000, "Data_Type"=enum."SGL", "Shift"=0.0, "Scale"=1.0} ("Input1D_Cfg"), "Size"=w15) -> (w18:T17)
  n8 = call-poly <vilib>:"NN_Layer_Create.vi"("Aug Config Params(1D)"=w17, "Input1D_Cfg"=w18, "error in (no error)"=w66, "NN in"=w67) -> ("error out"=w44:errorcluster, "NN out"=w43:T22)  [unwired: 5 in, 1 out]
  n9 = call-poly <vilib>:"NN_Layer_Create.vi"("FC_Cfg"=T12 {"Name"="FC_1", "Size"=2048, "BN"=FALSE, "BN_Params"={"epsilon"=0.0, "momentum"=0.0}, "Activation"=enum."Swish", "Has Bias?"=TRUE, "Init_Params"={"Init_Type"=enum."Xavier", "Value"=1.0}, "Custom_Params"=""} ("Layer_Config_Params"), "error in (no error)"=w44, "NN in"=w43) -> ("error out"=w39:errorcluster, "NN out"=w40:T22)  [unwired: 6 in, 1 out]
  n10 = call-poly <vilib>:"NN_Layer_Create.vi"("FC_Cfg"=T12 {"Name"="FC_2", "Size"=1024, "BN"=FALSE, "BN_Params"={"epsilon"=0.0, "momentum"=0.0}, "Activation"=enum."Swish", "Has Bias?"=TRUE, "Init_Params"={"Init_Type"=enum."Xavier", "Value"=1.0}, "Custom_Params"=""} ("Layer_Config_Params"), "error in (no error)"=w39, "NN in"=w40) -> ("error out"=w50:errorcluster, "NN out"=w51:T22)  [unwired: 6 in, 1 out]
  n11 = call-poly <vilib>:"NN_Layer_Create.vi"("FC_Cfg"=T12 {"Name"="FC_3", "Size"=512, "BN"=FALSE, "BN_Params"={"epsilon"=0.0, "momentum"=0.0}, "Activation"=enum."Swish", "Has Bias?"=TRUE, "Init_Params"={"Init_Type"=enum."Xavier", "Value"=1.0}, "Custom_Params"=""} ("Layer_Config_Params"), "error in (no error)"=w50, "NN in"=w51) -> ("error out"=w33:errorcluster, "NN out"=w34:T22)  [unwired: 6 in, 1 out]
  n12 = call-poly <vilib>:"NN_Layer_Create.vi"("FC_Cfg"=T12 {"Name"="FC_3", "Size"=256, "BN"=FALSE, "BN_Params"={"epsilon"=0.0, "momentum"=0.0}, "Activation"=enum."Swish", "Has Bias?"=TRUE, "Init_Params"={"Init_Type"=enum."Xavier", "Value"=1.0}, "Custom_Params"=""} ("Layer_Config_Params"), "error in (no error)"=w33, "NN in"=w34) -> ("error out"=w31:errorcluster, "NN out"=w32:T22)  [unwired: 6 in, 1 out]
  n13 = call-poly <vilib>:"NN_Layer_Create.vi"("FC_Cfg"=T12 {"Name"="FC_4", "Size"=10, "BN"=FALSE, "BN_Params"={"epsilon"=0.0, "momentum"=0.0}, "Activation"=enum."None", "Has Bias?"=TRUE, "Init_Params"={"Init_Type"=enum."Xavier", "Value"=1.0}, "Custom_Params"=""} ("Layer_Config_Params"), "error in (no error)"=w31, "NN in"=w32) -> ("error out"=w29:errorcluster, "NN out"=w30:T22)  [unwired: 6 in, 1 out]
  n14 = call-poly <vilib>:"NN_Layer_Create.vi"("FC_Cfg"=T12 {"Name"="FC_5", "Size"=256, "BN"=FALSE, "BN_Params"={"epsilon"=0.0, "momentum"=0.0}, "Activation"=enum."Swish", "Has Bias?"=TRUE, "Init_Params"={"Init_Type"=enum."Xavier", "Value"=1.0}, "Custom_Params"=""} ("Layer_Config_Params"), "error in (no error)"=w29, "NN in"=w30) -> ("error out"=w27:errorcluster, "NN out"=w28:T22)  [unwired: 6 in, 1 out]
  n15 = call-poly <vilib>:"NN_Layer_Create.vi"("FC_Cfg"=T12 {"Name"="FC_5", "Size"=512, "BN"=FALSE, "BN_Params"={"epsilon"=0.0, "momentum"=0.0}, "Activation"=enum."Swish", "Has Bias?"=TRUE, "Init_Params"={"Init_Type"=enum."Xavier", "Value"=1.0}, "Custom_Params"=""} ("Layer_Config_Params"), "error in (no error)"=w27, "NN in"=w28) -> ("error out"=w37:errorcluster, "NN out"=w38:T22)  [unwired: 6 in, 1 out]
  n16 = call-poly <vilib>:"NN_Layer_Create.vi"("FC_Cfg"=T12 {"Name"="FC_6", "Size"=1024, "BN"=FALSE, "BN_Params"={"epsilon"=0.0, "momentum"=0.0}, "Activation"=enum."Swish", "Has Bias?"=TRUE, "Init_Params"={"Init_Type"=enum."Xavier", "Value"=1.0}, "Custom_Params"=""} ("Layer_Config_Params"), "error in (no error)"=w37, "NN in"=w38) -> ("error out"=w45:errorcluster, "NN out"=w46:T22)  [unwired: 6 in, 1 out]
  n17 = Unbundle By Name(w2) -> ("Dims_Out"=w14:i32)
  n18 = call-poly <vilib>:"NN_Layer_Create.vi"("FC_Cfg"=T12 {"Name"="FC_7", "Size"=2048, "BN"=FALSE, "BN_Params"={"epsilon"=0.0, "momentum"=0.0}, "Activation"=enum."Swish", "Has Bias?"=TRUE, "Init_Params"={"Init_Type"=enum."Xavier", "Value"=1.0}, "Custom_Params"=""} ("Layer_Config_Params"), "error in (no error)"=w45, "NN in"=w46) -> ("error out"=w41:errorcluster, "NN out"=w42:T22)  [unwired: 6 in, 1 out]
  n19 = Bundle By Name(cluster=T12 {"Name"="Output", "Size"=2000, "BN"=FALSE, "BN_Params"={"epsilon"=0.0, "momentum"=0.0}, "Activation"=enum."None", "Has Bias?"=TRUE, "Init_Params"={"Init_Type"=enum."Xavier", "Value"=1.0}, "Custom_Params"=""} ("Layer_Config_Params"), "Size"=w14) -> (w16:T12)
  n20 = call-poly <vilib>:"NN_Layer_Create.vi"("FC_Cfg"=w16, "error in (no error)"=w41, "NN in"=w42) -> ("error out"=w24:errorcluster, "NN out"=w62:T22)  [unwired: 6 in, 1 out]
  n21 = call-poly <vilib>:"NN_Set_Loss.vi"("error in (no error)"=w24, "NN in"=w62) -> ("error out"=w23:errorcluster, "NN out"=w25:T22)  [unwired: 8 in]
  n22 = Unbundle By Name(w1) -> ("Dataset_Size"=w13:i32)
  n23 = call-poly <vilib>:"NN_Check_Dataset.vi"("Dataset"=w2, "error in (no error)"=w23, "NN in"=w25) -> ("error out"=w55:errorcluster, "NN out"=w56:T22)  [unwired: 7 in]
  n24 = Decrement(x=w13) -> (x-1=w22:i32)
  n25 = call <vilib>:"NN_Set_Train_Config.vi"("NN_Train_Params"="Train_Params", "error in (no error)"=w55, "NN in"=w56) -> ("error out"=w60:errorcluster, "NN out"=w61:T22)  [unwired: 7 in]
  n26 = property on="Sample Index" class="DigNum (strict)"("Maximum"=w22, "Minimum"=0.0 ("Data Entry Limits:Minimum")) -> ()  [unwired: 2 in, 2 out]
  n27 = flat-sequence {
    tunnel: [w69] -> w65
    tunnel: w60 -> [_]
    frame #0 {
      n28 = call <vilib>:"High Resolution Relative Seconds.vi"() -> ("relative seconds"=w69:dbl)
    }
  }
  n29 = while {
    shift-right: [w82] -> w11
    shift-left: w60 -> [w85]
    shift-right: [w81] -> w12
    shift-left: w61 -> [w86]
    tunnel: w65 -> [w91]
    tunnel: w2 -> [w80]
    tunnel: w3 -> [w72]
    tunnel: w1 -> [w71]
    stop <- w94 stop-if-true
    n30 = call <vilib>:"NN_Cfg_LR_Decay_Policy.vi"("LR_Decay_Params"="LR Update Policy", "error in (no error)"=w85, "NN in"=w86) -> ("error out"=w92:errorcluster, "NN out"=w95:T22)  [unwired: 7 in]
    n31 = call <vilib>:"High Resolution Relative Seconds.vi"() -> ("relative seconds"=w90:dbl)
    n32 = call <vilib>:"NN_Train.vi"("Train Dataset"=w80, "error in (no error)"=w92, "NN in"=w95) -> ("error out"=w83:errorcluster, "NN out"=w84:T22, "Loss"=w93:sgl)  [unwired: 3 in, 3 out]
    n33 = feedback #1() -> (w96:dbl)  [unwired: 1 in]
    n34 = feedback-in #1(w90) -> ()
    n35 = Unbundle By Name(w84) -> ("Session Data"=→"Session Data":T1)
    n36 = Unbundle By Name(w86) -> ("mBatch"=w88:i32)
    n37 = Compound Arithmetic op=OR(w83, "Stop") -> (w94:bool)
    n38 = call <vilib>:"Running_AVG_FIR_Filter.vi"("Numeric"=w93) -> ("Filtered x"=→"Train Loss" →"Loss Chart":sgl)  [unwired: 10 in]
    n39 = Subtract(x=w90, y=w91) -> (x-y=→"Time_Elapsed":dbl)
    n40 = Subtract(x=w90, y=w96) -> (x-y=w78:dbl)
    "Train Speed (sec/iter)" <- w78
    n41 = Select(t=w71, s="Normal/Abnormal", f=w72) -> (s? t:f=w70:T20)
    n42 = case shown="True" "Check?" {
      tunnel: w84 -> [w98 w118]
      tunnel: w83 -> [w97 w126]
      tunnel: [w97 w125] -> w82
      tunnel: [w98 w104] -> w81
      tunnel: w70 -> [_ w111]
      frame False {
      }
      frame True {
        w112 = sgl 240.0 ("x")
        n43 = Unbundle By Name(w111) -> ("Inputs Ref."=w101:variant)
        n44 = Bundle By Name(cluster=w118, "Train?"=FALSE) -> (w119:T22)
        n45 = call-poly <vilib>:"NN_Data_Variant_to_DVR.vi"("error in (no error)"=w126, "Inputs Ref."=w101) -> ("error out"=w100:errorcluster, "DVR(2D_SGL)"=w99:T21)  [unwired: 8 in]
        n46 = call-poly <vilib>:"NN_Data_Get_ValByRef.vi"("index (row)"="Sample Index", "DVR(2D_SGL)"=w99) -> ("Value(1D_SGL)"=w102:sgl[])  [unwired: 6 in, 1 out]
        n47 = call-poly <vilib>:"NN_Set_Input.vi"("error in (no error)"=w100, "Data_In(1D_SGL)"=w102, "NN In"=w119) -> ("error out"=w121:errorcluster, "NN Out"=w120:T22)  [unwired: 7 in]
        n48 = call <vilib>:"NN_Forward.vi"("error in (no error)"=w121, "NN in"=w120) -> ("error out"=w123:errorcluster, "NN out"=w124:T22)  [unwired: 6 in, 2 out]
        n49 = call <vilib>:"NN_Get_Layer(Last).vi"("error in (no error)"=w123, "NN in"=w124) -> ("error out"=w116:errorcluster, "Last_Layer"=w117:T32, "NN out"=w114:T22)  [unwired: 6 in, 1 out]
        n50 = call <vilib>:"NN_Layer_Get_OutVals_as1D.vi"("error in (no error)"=w116, "Layer"=w117) -> ("error out"=w125:errorcluster, "Out(as1D)"=w115:sgl[][])  [unwired: 8 in]
        n51 = Index Array(array=w115) -> (element=w103:sgl[])  [unwired: 2 in]
        n52 = Subtract(x=w102, y=w103) -> (x-y=w109:sgl[])
        n53 = Absolute Value(x=w109) -> (abs(x)=→"Anomaly Score":sgl[])
        n54 = Multiply(x=w103, y=w112) -> (x*y=w110:sgl[])
        n55 = Multiply(x=w102, y=w112) -> (x*y=w108:sgl[])
        n56 = Bundle By Name(cluster=w114, "Train?"=TRUE) -> (w104:T22)
        n57 = Build Array(w110, w108) -> (→"Input & Reconstructed Signals":sgl[][])
      }
    }
    n58 = Divide(x=w88, y=w78) -> (x/y=→"Train Speed (Sample/sec)":dbl)
  }
  n59 = call <vilib>:"NN_Destroy.vi"("Save (T, T, T)"=T19 {"CFG?"=TRUE, "Weights?"=TRUE, "Render?"=TRUE} ("Save_Config"), "error in (no error)"=w11, "NN in"=w12) -> ()  [unwired: 7 in, 2 out]
